vi "Facade.vi"(0 "Data In":T38, 2 "Display State In":T11, 3 "Container State":T37) -> (6 "Data Out":T38, 7 "Display State Out":T11, 8 "Action":T10)   [LabVIEW 2020, in "3DPC_SurfacePlot.xctl"]
uses:
  <vilib>/Native 3D Graph/xcontrol/3DPC_SurfacePlot.xctl
  <vilib>/Native 3D Graph/xcontrol/Data.ctl
  <vilib>/Native 3D Graph/classes/Base Datatype.lvclass
  <vilib>/_xctls/Container State.ctl
  <vilib>/Native 3D Graph/xcontrol/State.ctl
  <vilib>/Native 3D Graph/typedefs/prop_graph.ctl
  <vilib>/Native 3D Graph/typedefs/all_non_graph_prop.ctl
  <vilib>/Native 3D Graph/typedefs/prop_plot_all_array.ctl
  <vilib>/Native 3D Graph/typedefs/prop_plot_all.ctl
  <vilib>/Native 3D Graph/typedefs/prop_plot_projection.ctl
  <vilib>/Native 3D Graph/typedefs/prop_plot_surface.ctl
  <vilib>/Native 3D Graph/typedefs/prop_plot_contour.ctl
  <vilib>/Native 3D Graph/typedefs/prop_plot_normal.ctl
  <vilib>/Native 3D Graph/typedefs/prop_plot_point_line.ctl
  <vilib>/Native 3D Graph/typedefs/prop_value_pair_all.ctl
  <vilib>/Native 3D Graph/typedefs/prop_value_pair_1d.ctl
  <vilib>/Native 3D Graph/typedefs/prop_axes_all.ctl
  <vilib>/Native 3D Graph/typedefs/prop_axes_grid.ctl
  <vilib>/Native 3D Graph/typedefs/prop_axes_ticks.ctl
  <vilib>/Native 3D Graph/typedefs/range_cluster.ctl
  <vilib>/Native 3D Graph/typedefs/min_max.ctl
  <vilib>/Native 3D Graph/typedefs/prop_axes_captions.ctl
  <vilib>/Native 3D Graph/typedefs/prop_axes_labels.ctl
  <vilib>/Native 3D Graph/typedefs/prop_axes_autorange.ctl
  <vilib>/Native 3D Graph/typedefs/prop_cursor_all_array.ctl
  <vilib>/Native 3D Graph/typedefs/prop_cursor_point.ctl
  <vilib>/Native 3D Graph/typedefs/prop_cursor_position.ctl
  <vilib>/Native 3D Graph/typedefs/prop_cursor_line.ctl
  <vilib>/Native 3D Graph/typedefs/prop_cursor_plane.ctl
  <vilib>/Native 3D Graph/typedefs/prop_cursor_text.ctl
  <vilib>/Native 3D Graph/typedefs/prop_format.ctl
  <vilib>/Native 3D Graph/typedefs/prop_lighting.ctl
  <vilib>/_xctls/Action.ctl
  <vilib>/Native 3D Graph/xcontrol/Processed Data.ctl
  <vilib>/Native 3D Graph/typedefs/plot_rep_array.ctl
  <vilib>/Native 3D Graph/typedefs/plot_rep.ctl
  <vilib>/Native 3D Graph/typedefs/plot_rep_mesh_data.ctl
  <vilib>/Native 3D Graph/typedefs/prop_axes_merged_array_etc.ctl
  <vilib>/Native 3D Graph/typedefs/prop_axes_merged_array.ctl
  <vilib>/Utility/miscctls.llb/LVRectTypeDef.ctl
  <vilib>/Native 3D Graph/typedefs/track_eye.ctl
  <vilib>/Native 3D Graph/typedefs/vector.ctl
  <vilib>/Native 3D Graph/typedefs/update_scene_all.ctl
  <vilib>/Native 3D Graph/typedefs/update_scene_component.ctl
  <vilib>/Utility/miscctls.llb/LVPoint32TypeDef.ctl
  <vilib>/picture/3D Picture Control/Object/Create Object (name).vi
  <vilib>/_xctls/XControlSupport.lvlib
  <vilib>/picture/3D Picture Control/NI_3D Picture Control.lvlib
panel:
  in  "Last Axis output cluster":T1={"X Merged Array"=[], "Y Merged Array"=[], "Z Merged Array"=[], "Range Min/Max"={"X"={"Min"=0.0, "Max"=0.0}, "Y"={"Min"=0.0, "Max"=0.0}, "Z"={"Min"=0.0, "Max"=0.0}, "Amplitude"={"Min"=-123456.0, "Max"=-123456.0}}}
  in  "String 2":string="Render Window"
  in  "String":string="3D Graph Properties"
  in  "Coord Systems":T5(array[ring])=[enum."Spherical"]
  in  "Dummy":bool=TRUE
  out "Plot processed data out":T6={"Plot Rep Arrays"=[], "Graph Range Min/Max"={"X"={"Min"=0.0, "Max"=-inf}, "Y"={"Min"=0.0, "Max"=-inf}, "Z"={"Min"=inf, "Max"=-inf}, "Amplitude"={"Min"=0.0, "Max"=0.0}}}
  in  "Plot processed data In":T6={"Plot Rep Arrays"=[], "Graph Range Min/Max"={"X"={"Min"=0.0, "Max"=-inf}, "Y"={"Min"=0.0, "Max"=-inf}, "Z"={"Min"=inf, "Max"=-inf}, "Amplitude"={"Min"=0.0, "Max"=0.0}}} caption="Data In"
  out "Hardware Window Refnum":refnum<vi>
  out "3D Picture Control":refnum<vi>(3d-picture)
types:
  T1 = typedef "3DPC_SurfacePlot.xctl/prop_axes_merged_array_etc.ctl" = cluster{"X Merged Array":T2, "Y Merged Array":T2, "Z Merged Array":T2, "Range Min/Max":T3}
  T2 = typedef "3DPC_SurfacePlot.xctl/prop_axes_merged_array.ctl" = cluster{"Show Tick":bool, "Show Line":bool, "Interval":sgl, "Name":string}[]
  T3 = typedef "3DPC_SurfacePlot.xctl/range_cluster.ctl" = cluster{"X":T4, "Y":T4, "Z":T4, "Amplitude":T4}
  T4 = typedef "3DPC_SurfacePlot.xctl/min_max.ctl" = cluster{"Min":sgl, "Max":sgl}
  T5 = enum16{"Cartesian", "Cylindrical", "Spherical"}[]
  T6 = typedef "Processed Data.ctl" = cluster{"Plot Rep Arrays":T7, "Graph Range Min/Max":T3}
  T7 = typedef "3DPC_SurfacePlot.xctl/plot_rep_array.ctl" = T8[]
  T8 = typedef "3DPC_SurfacePlot.xctl/plot_rep.ctl" = cluster{"Plot ID":i32, "Plot Range Min/Max Out":T3, "Mesh Data":T9}
  T9 = typedef "3DPC_SurfacePlot.xctl/plot_rep_mesh_data.ctl" = cluster{"Index Array":u32[], "Normal Array":cluster{"X":sgl, "Y":sgl, "Z":sgl}[], "Vertex Array":cluster{"X":sgl, "Y":sgl, "Z":sgl}[], "Draw Mode":enum16{"Points", "Lines", "Line Strip", "Line Loop", "Triangles", "Triangle Strip", "Triangle Fan", "Quads", "Quad Strip", "Polygon"}, "Coordinate System":enum16{"Cartesian", "Cylindrical", "Spherical"}, "Color Index Array":i32[]}
  T10 = typedef "XControlSupport.lvlib/Action.ctl" = cluster{"Data Changed?":bool, "State Changed?":bool, "Action Name":string}
  T11 = typedef "3DPC_SurfacePlot.xctl/State.ctl" = cluster{"Graph Properties":T12, "Plot/Axes/Cursor Properties":T13, "Active Plot":i32, "Active Axis":i32, "Active Cursor":i32, "Disable Updates":bool}
  T12 = typedef "3DPC_SurfacePlot.xctl/prop_graph.ctl" = cluster{"Projection Mode":enum16{"Orthographic", "Perspective"}, "View Direction":enum32{"Towards X-Y Plane", "Towards Y-Z Plane", "Towards X-Z Plane", "User Define"}, "Plot Area Color":u32, "Fast Draw":bool, "X-Y":bool, "Y-Z":bool, "X-Z":bool, "Lighting":bool, "Refnum Queue":refnum<queue>}
  T13 = typedef "3DPC_SurfacePlot.xctl/all_non_graph_prop.ctl" = cluster{"Plot Properties Array":T14, "Value Pair Properties":T21, "Axes Properties":T23, "Cursor Properties Array":T29, "Format strings":T35, "Lighting Properties":T36, "Lights":cluster{"Position":cluster{"X":sgl, "Y":sgl, "Z":sgl}, "Direction":cluster{"X":sgl, "Y":sgl, "Z":sgl}}[]}
  T14 = typedef "3DPC_SurfacePlot.xctl/prop_plot_all_array.ctl" = T15[]
  T15 = typedef "3DPC_SurfacePlot.xctl/prop_plot_all.ctl" = cluster{"Projection Properties":T16, "Surface Properties":T17, "Contour Properties":T18, "Normal Properties":T19, "Points/Lines Properties":T20, "Plot ID":i32, "Coordinate System":enum16{"Cartesian", "Cylindrical", "Spherical"}}
  T16 = typedef "3DPC_SurfacePlot.xctl/prop_plot_projection.ctl" = cluster{"Draw XY":bool, "Draw YZ":bool, "Draw XZ":bool}
  T17 = typedef "3DPC_SurfacePlot.xctl/prop_plot_surface.ctl" = cluster{"Draw surface":bool, "Opacity":dbl, "Shading":bool, "Specular":i32, "Color Map":cluster{dbl, u32}[], "Interpolate Color":bool, "Absolute Colormap":bool}
  T18 = typedef "3DPC_SurfacePlot.xctl/prop_plot_contour.ctl" = cluster{"Contour color":u32, "Axis":enum16{"X", "Y", "Z"}, "Draw contour":bool, "Antialias":bool, "Line Width":sgl, "Contour Line Style":enum16{"Solid", "Dash", "Dot", "Dash Dot"}, "Mode":enum16{"Levels", "Intervals", "Level List"}, "Levels":sgl, "Intervals":sgl, "Anchored At":sgl, "Anchored":bool, "Level List":dbl[]}
  T19 = typedef "3DPC_SurfacePlot.xctl/prop_plot_normal.ctl" = cluster{"Normal color":u32, "Normal Length":sgl, "Normal Width":sgl, "Draw Normal":bool, "Antialiasing":bool}
  T20 = typedef "3DPC_SurfacePlot.xctl/prop_plot_point_line.ctl" = cluster{"Color":u32, "Antialiasing":bool, "Point Size":sgl, "Points / Lines":enum16{"None", "Points", "Lines", "Both"}, "Point Style":enum16{"Point", "EmptySquare", "Asterisk", "Diamond", "EmptyCircle", "Circle", "X"}, "Line Style":enum16{"Solid", "Dash", "Dot", "Dash Dot"}, "Line Width":sgl}
  T21 = typedef "3DPC_SurfacePlot.xctl/prop_value_pair_all.ctl" = cluster{"X Value Pairs":cluster{"Data Array":cluster{"Value":sgl, "Index":i32, "Name":string}[], "Show ticks":bool, "Show grid lines":bool, "Labels":enum16{"Value", "None", "Name"}}, "Y Value Pairs":T22, "Z Value Pairs":T22}
  T22 = typedef "3DPC_SurfacePlot.xctl/prop_value_pair_1d.ctl" = cluster{"Data Array":cluster{"Value":sgl, "Index":i32, "Name":string}[], "Show ticks":bool, "Show grid lines":bool, "Labels":enum16{"Value", "None", "Name"}}
  T23 = typedef "3DPC_SurfacePlot.xctl/prop_axes_all.ctl" = cluster{"Grid  Properties":T24, "Ticks Properties":T25, "from/to cluster":T3, "Caption Properties":T26, "Labels Properties":T27, "Auto Range On":T28}
  T24 = typedef "3DPC_SurfacePlot.xctl/prop_axes_grid.ctl" = cluster{"Grid Visible":cluster{"Draw X-grid":bool, "Draw Y-grid":bool, "Draw Z-grid":bool}, "Grid Color":cluster{"Color X":u32, "Color Y":u32, "Color Z":u32}}
  T25 = typedef "3DPC_SurfacePlot.xctl/prop_axes_ticks.ctl" = cluster{"Minor Count":cluster{"X":i32, "Y":i32, "Z":i32}, "Major Count":cluster{"X":i32, "Y":i32, "Z":i32}, "Major Ticks Visible":cluster{"X":bool, "Y":bool, "Z":bool}, "Minor Ticks Visible":cluster{"X":bool, "Y":bool, "Z":bool}, "Tick Color":cluster{"Color X":u32, "Color Y":u32, "Color Z":u32}}
  T26 = typedef "3DPC_SurfacePlot.xctl/prop_axes_captions.ctl" = cluster{"Show Captions":cluster{"Show X Caption":bool, "Show Z Caption":bool, "Show Y Caption":bool, "Show Opposite X Caption":bool, "Show Opposite Y Caption":bool, "Show Opposite Z Caption":bool}, "Captions":cluster{"Caption X":string, "Caption Y":string, "Caption Z":string}, "Caption Color":cluster{"Color X":u32, "Color Y":u32, "Color Z":u32}, "Caption Font Size":cluster{"Font Size X":i16, "Font Size Y":i16, "Font Size Z":i16}}
  T27 = typedef "3DPC_SurfacePlot.xctl/prop_axes_labels.ctl" = cluster{"Label Visible":cluster{"Show X Labels":bool, "Show Y Labels":bool, "Show Z Labels":bool, "Show Opposite X Labels":bool, "Show Opposite Y Labels":bool, "Show Opposite Z Labels":bool}, "Label Color":cluster{"Color X":u32, "Color Y":u32, "Color Z":u32}, "Label Font Size":cluster{"Font Size X":i16, "Font Size Y":i16, "Font Size Z":i16}}
  T28 = typedef "3DPC_SurfacePlot.xctl/prop_axes_autorange.ctl" = cluster{"X":bool, "Y":bool, "Z":bool}
  T29 = typedef "3DPC_SurfacePlot.xctl/prop_cursor_all_array.ctl" = cluster{"Cursor Visible":bool, "Cursor Enable":bool, "Cursor Point":T30, "Cursor Position":T31, "Cursor Line":T32, "Cursor Plane":T33, "Cursor Name":string, "Cursor Text":T34}[]
  T30 = typedef "3DPC_SurfacePlot.xctl/prop_cursor_point.ctl" = cluster{"Point Color":u32, "Point Size":dbl, "Point Visible":bool}
  T31 = typedef "3DPC_SurfacePlot.xctl/prop_cursor_position.ctl" = cluster{"Position X":dbl, "Position Y":dbl, "Position Z":dbl, "Position Snap To":enum16{"Fixed", "Nearest Plot", "Snap to Plot"}, "Polsition Pick Plot":u16, "Position Column":i32, "Position Row":i32}
  T32 = typedef "3DPC_SurfacePlot.xctl/prop_cursor_line.ctl" = cluster{"Line Color":u32, "Line Width":dbl, "Line Visible":bool}
  T33 = typedef "3DPC_SurfacePlot.xctl/prop_cursor_plane.ctl" = cluster{"Plane Opacity":dbl, "Plane Color":u32, "Plane YZ":bool, "Plane XZ":bool, "Plane XY":bool}
  T34 = typedef "3DPC_SurfacePlot.xctl/prop_cursor_text.ctl" = cluster{"Cursor Name":string, "Font Size":i32, "Show Position":bool, "Show Name":bool, "Text Color":u32, "Back Color":u32, "Opacity":dbl}
  T35 = typedef "3DPC_SurfacePlot.xctl/prop_format.ctl" = cluster{"XAxis":string, "YAxis":string, "ZAxis":string}
  T36 = typedef "3DPC_SurfacePlot.xctl/prop_lighting.ctl" = cluster{"Brightness":i32, "Focus":dbl, "Linear Attenuation":dbl, "Quadratic Attenuation":dbl}
  T37 = typedef "XControlSupport.lvlib/Container State.ctl" = cluster{"Indicator?":bool, "Run Mode?":bool, " Refnum":refnum<vi>}
  T38 = typedef "3DPC_SurfacePlot.xctl/Data.ctl" = refnum<class "Base Datatype.lvclass">[]
  T39 = typedef "3DPC_SurfacePlot.xctl/track_eye.ctl" = cluster{"Forward Vect":T40, "Up Vect":T40}
  T40 = typedef "3DPC_SurfacePlot.xctl/vector.ctl" = cluster{"X":sgl, "Y":sgl, "Z":sgl}
  T41 = typedef "LVRectTypeDef.ctl" = cluster{"Left":i16, "Top":i16, "Right":i16, "Bottom":i16}
  T42 = enum16{"Open", "Minimized", "Maximized", "Hidden"}
  T43 = typedef "3DPC_SurfacePlot.xctl/update_scene_all.ctl" = cluster{"Update Plot":T44, "Update Grid":T44, "Update Cursor":T44, "Update Fast Draw":T44}
  T44 = typedef "3DPC_SurfacePlot.xctl/update_scene_component.ctl" = enum16{"Update & Add", "Update & Not Add", "Remove ", "Nothing", "Add"}
  T45 = enum32{"Towards X-Y Plane", "Towards Y-Z Plane", "Towards X-Z Plane", "User Define"}
  T46 = typedef "LVPoint32TypeDef.ctl" = cluster{"Horizontal":i32, "Vertical":i32}
  T47 = cluster{"Real Matrix Element":dbl, "Real Matrix Element":dbl, "Real Matrix Element":dbl}[]
  T48 = cluster{"Left":sgl, "Left":sgl, "Left":sgl, "Left":sgl, "Left":sgl, "Left":sgl}
  T49 = enum16{"None", "Spherical", "Flying", "Oriented"}
  T50 = cluster{"Position":cluster{"X":sgl, "Y":sgl, "Z":sgl}, "Direction":cluster{"X":sgl, "Y":sgl, "Z":sgl}}[]
  T51 = typedef "LVBoundsTypeDef.ctl" = cluster{"Width":u32, "Height":u32}
  T52 = typedef "3DPC_SurfacePlot.xctl/state_scene_objects.ctl" = cluster{"Root":refnum<vi>, "Fast Draw Scene Object":refnum<vi>, "Plot Scene Object":refnum<vi>, "Axes Scene Object":refnum<vi>, "Cursor Scene Object":refnum<vi>, "PL Scene Object":refnum<vi>}
  T53 = cluster{"Cursor Visible":bool, "Cursor Enable":bool, "Cursor Point":T30, "Cursor Position":T31, "Cursor Line":T32, "Cursor Plane":T33, "Cursor Name":string, "Cursor Text":T34}
  T54 = typedef "LV3DPointTypeDef.ctl" = cluster{"X":sgl, "Y":sgl, "Z":sgl}
  T55 = cluster{"X":cluster{"Min":bool, "Max":bool}, "Y":cluster{"Min":bool, "Max":bool}, "Z":cluster{"Min":bool, "Max":bool}, "Amplitude":cluster{"Min":bool, "Max":bool}}
  T56 = cluster{"Shift":bool, "Ctrl":bool, "Alt":bool, "Cmd":bool, "Opt":bool}
  T57 = cluster{"Position X":dbl, "Position Y":dbl, "Position Z":dbl}
  T58 = cluster{"Position X":dbl, "Position Y":dbl, "Position Z":dbl}[]
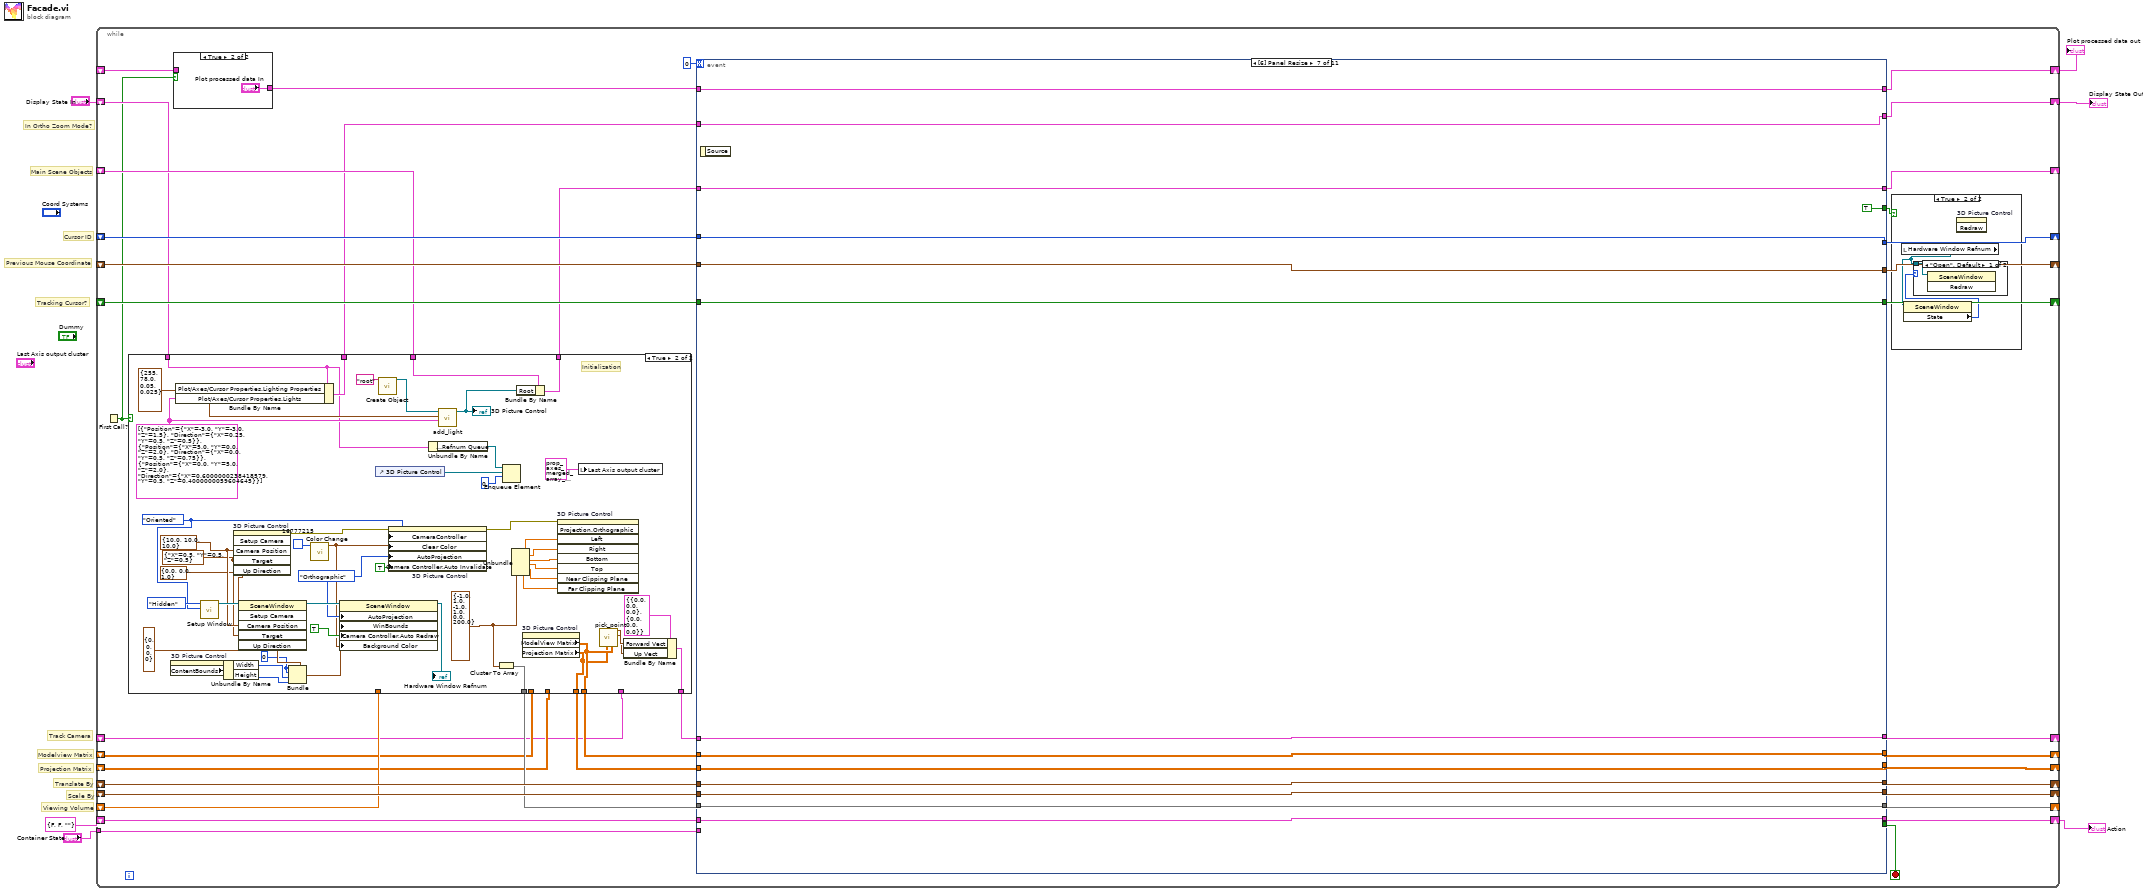
[diagram p0: block diagram]
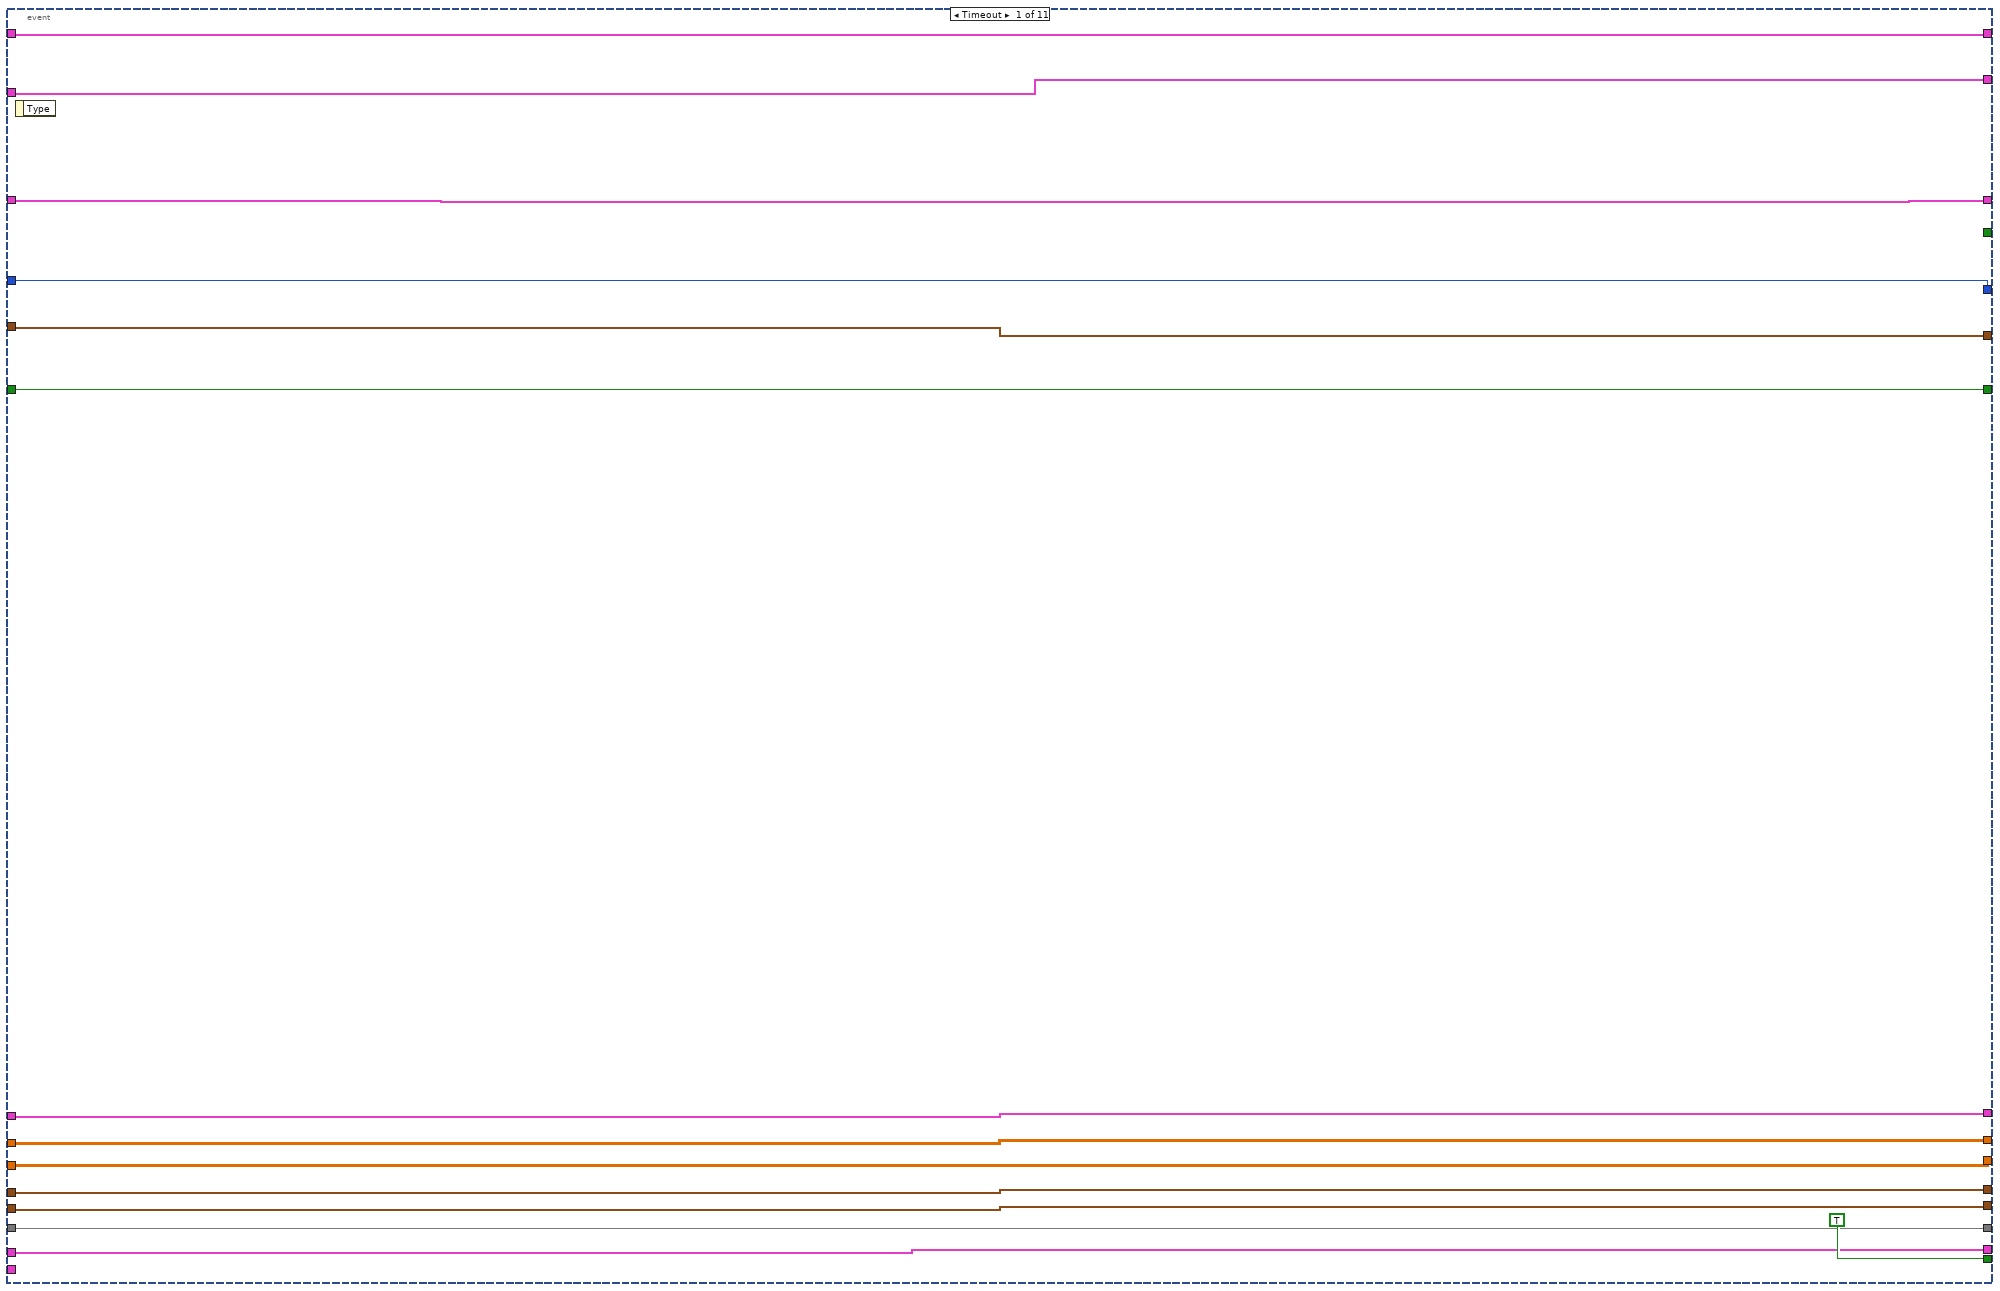
[diagram p6: hidden frame]
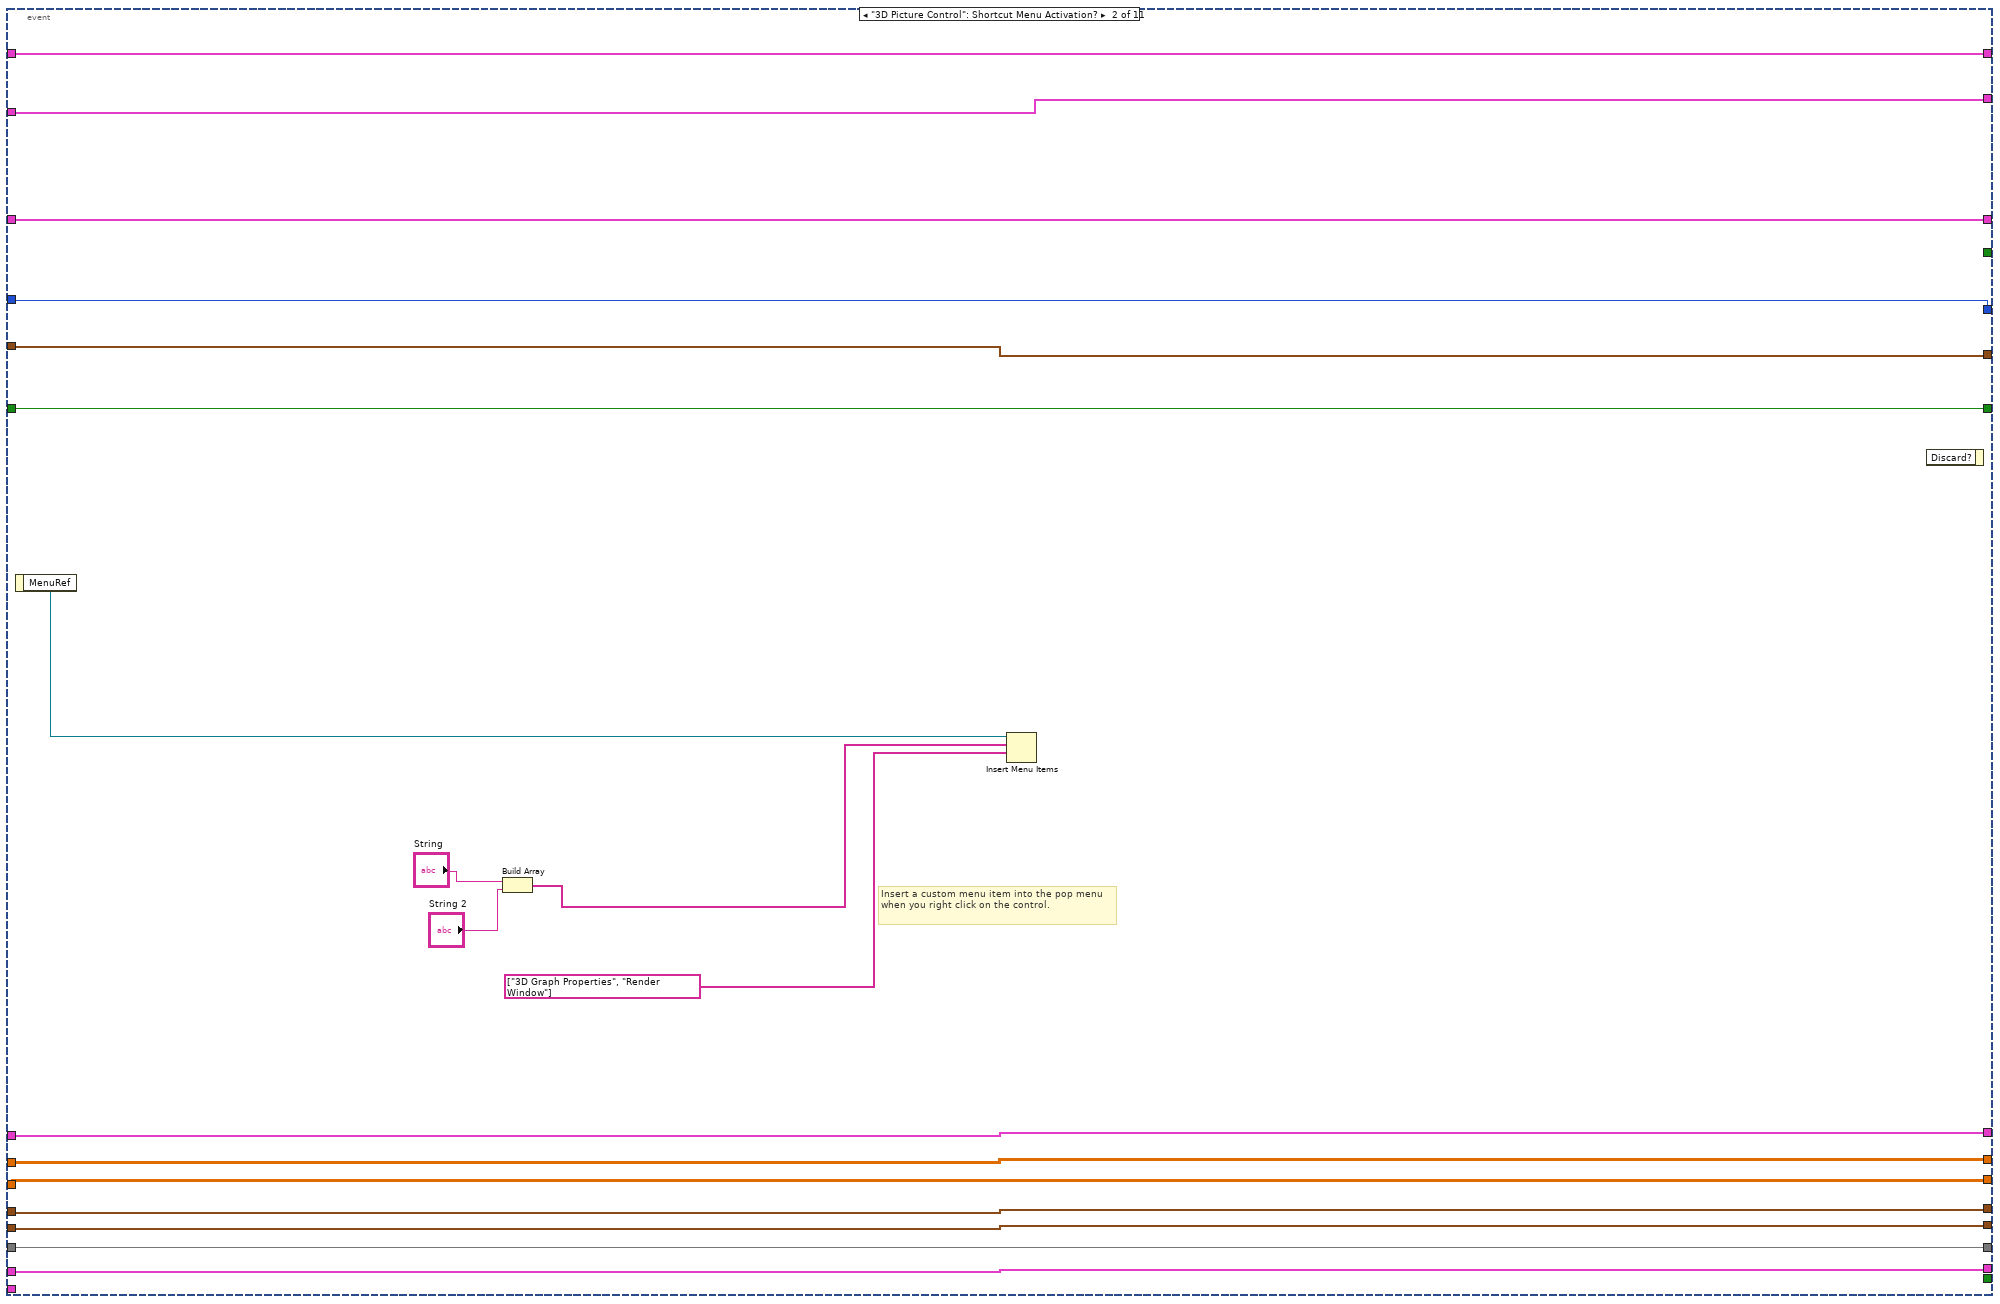
[diagram p7: hidden frame]
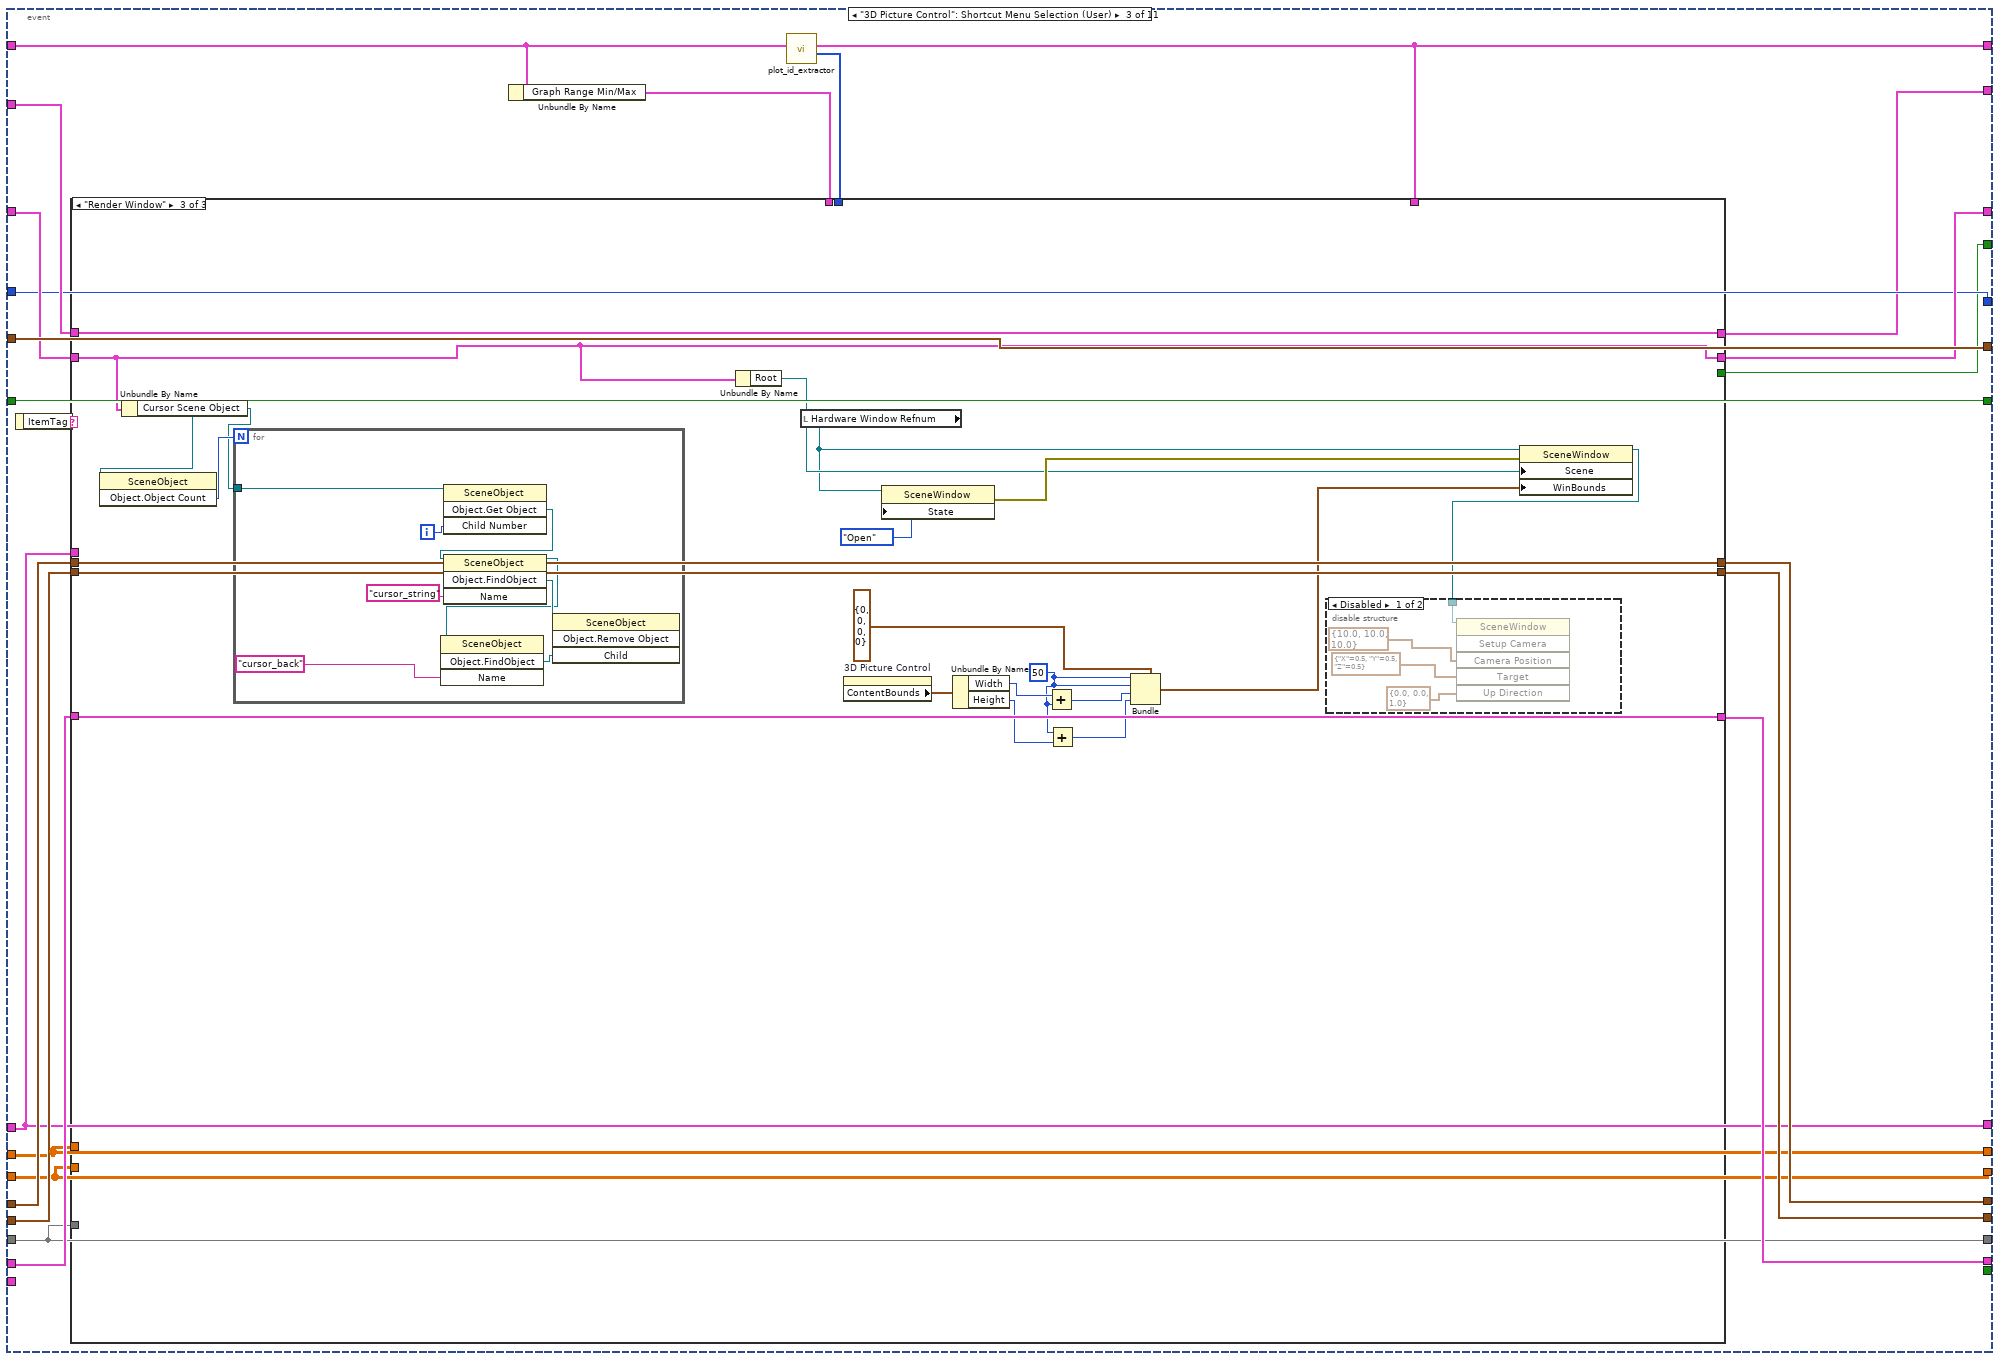
[diagram p8: hidden frame]
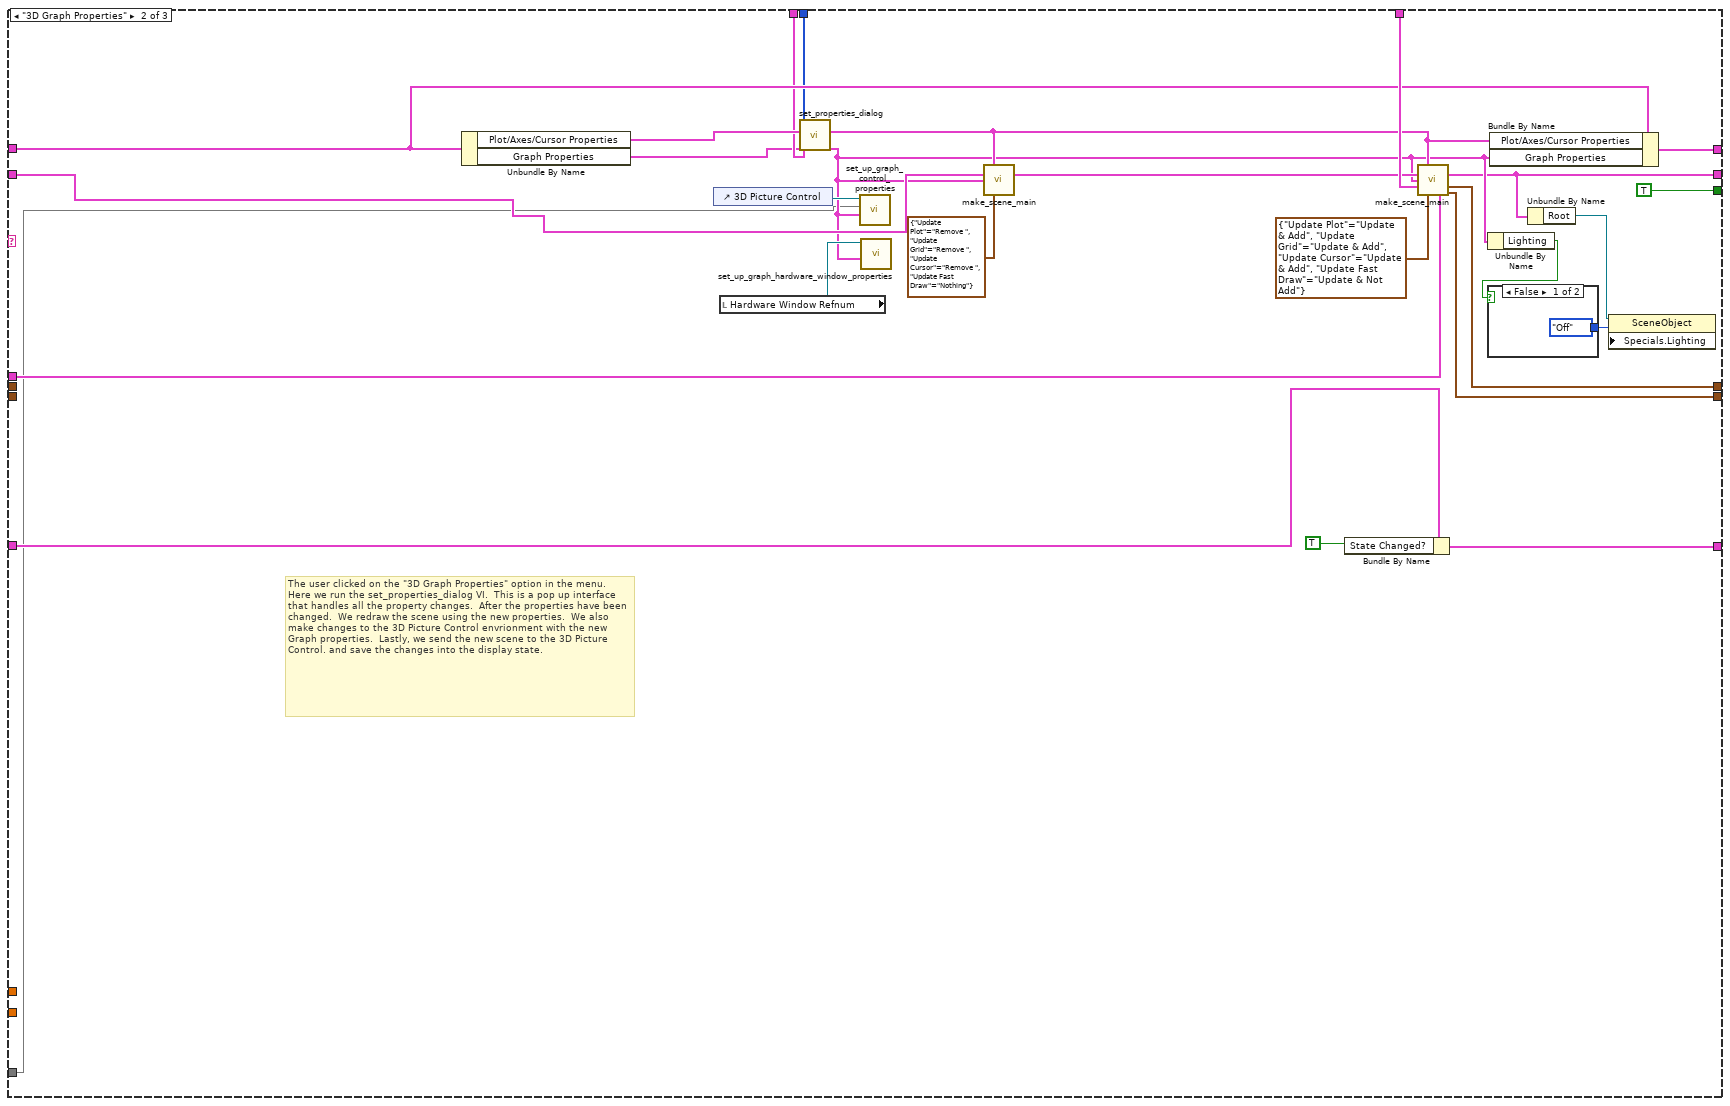
[diagram p10: hidden frame]
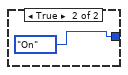
[diagram p11: hidden frame]
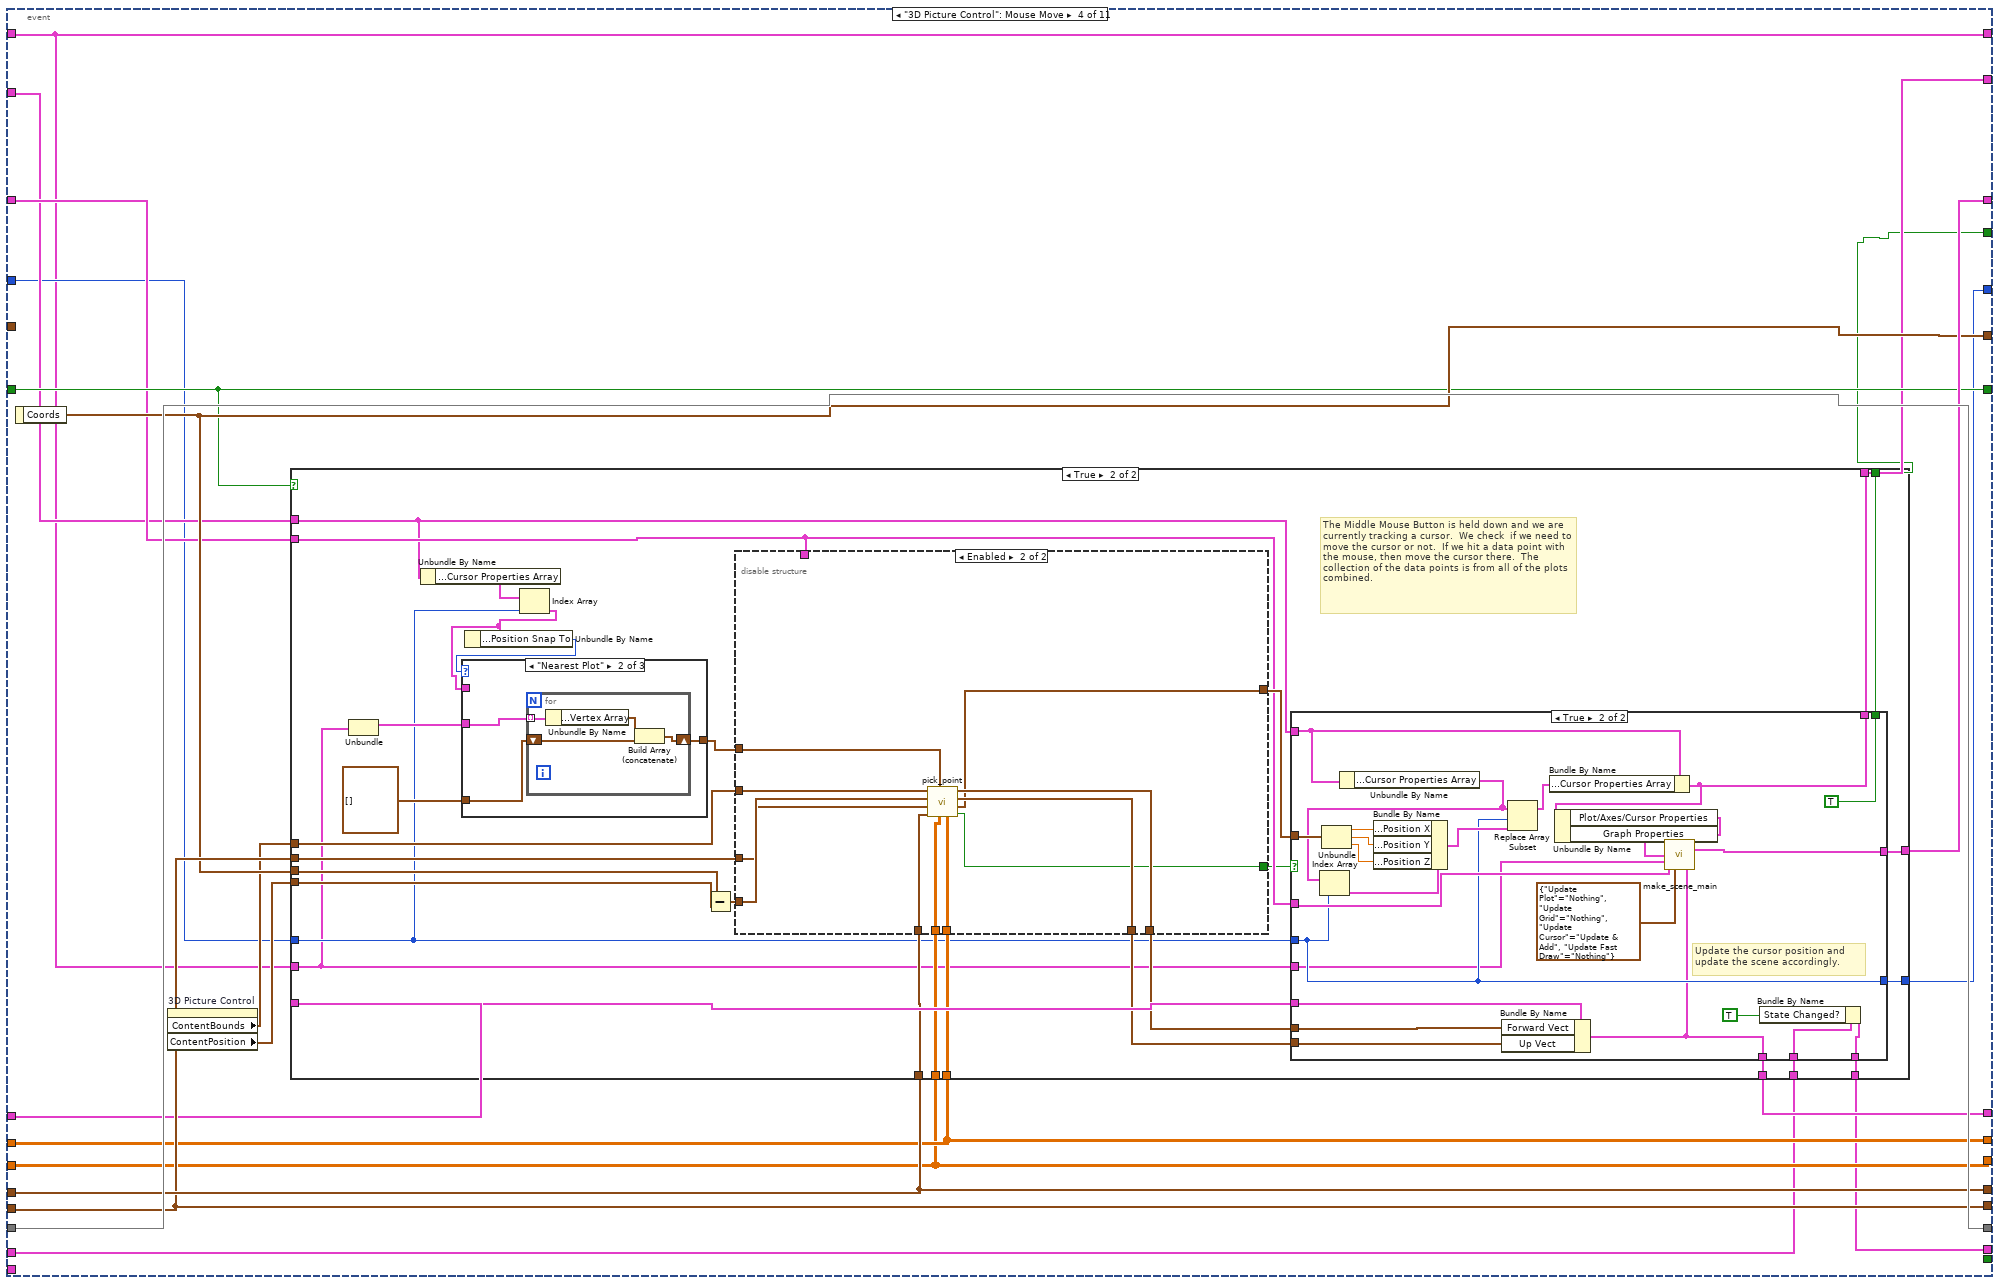
[diagram p13: hidden frame]
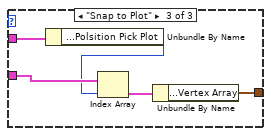
[diagram p16: hidden frame]
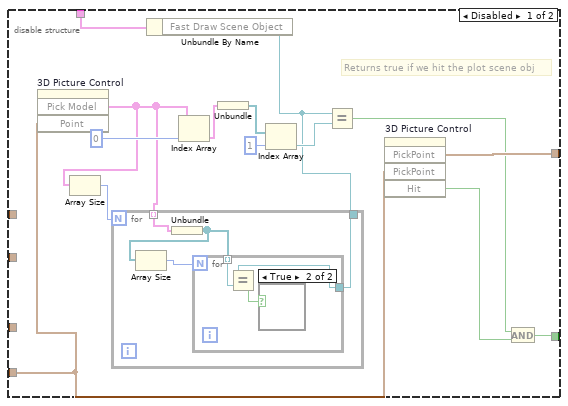
[diagram p17: hidden frame]
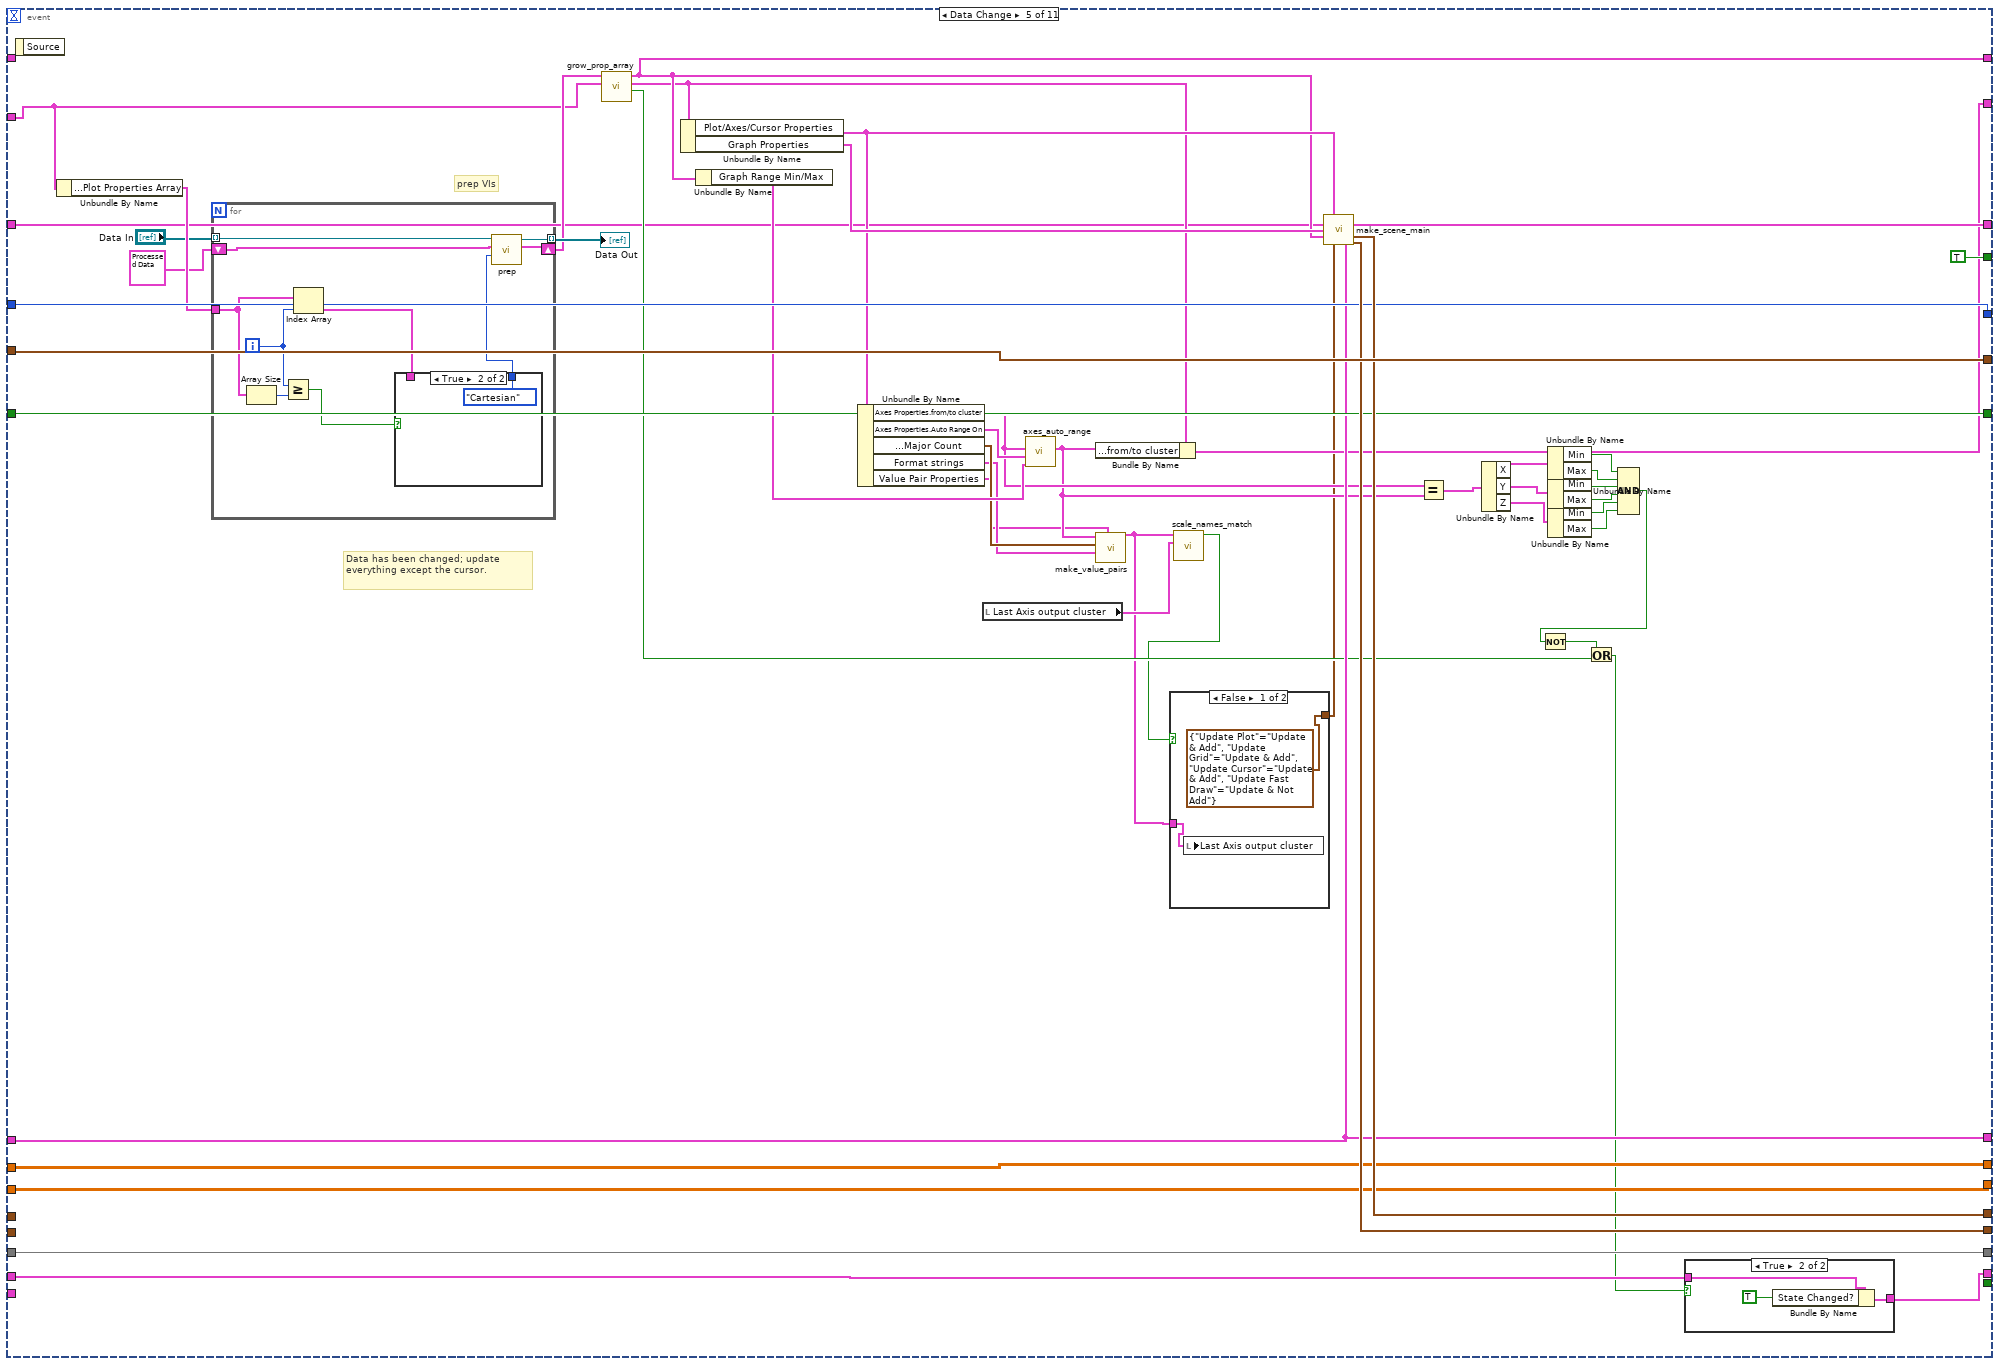
[diagram p20: hidden frame]
diagram:
  # "Viewing Volume"
  # "Main Scene Objects"
  # "Cursor ID"
  # "Scale By"
  # "Translate By"
  # "Projection Matrix"
  # "Modelview Matrix"
  # "Track Camera"
  # "Tracking Cursor?"
  # "In Ortho Zoom Mode?"
  # "Previous Mouse Coordinate"
  n1 = while {
    shift-right: [w25] -> w3
    shift-left: "Display State In" -> [w18]
    tunnel: "Container State" -> [w42]
    shift-right: [w16] -> w6
    shift-left: _ -> [w14]
    shift-right: [w40] -> w4
    shift-left: T10 {"Data Changed?"=FALSE, "State Changed?"=FALSE, "Action Name"=""} ("Action") -> [w41]
    shift-right: [w38] -> _
    shift-left: _ -> [w39]
    shift-right: [w37] -> _
    shift-left: _ -> [w21]
    shift-right: [w36] -> _
    shift-left: _ -> [w24]
    shift-right: [w26] -> _
    shift-left: _ -> [w28]
    shift-right: [w31] -> _
    shift-left: _ -> [w8]
    shift-right: [w30] -> _
    shift-left: _ -> [w12]
    shift-right: [w35] -> _
    shift-left: _ -> [w33]
    shift-right: [w34] -> _
    shift-left: _ -> [w32]
    shift-right: [w27] -> _
    shift-left: _ -> [w29]
    shift-right: [w19] -> _
    shift-left: _ -> [w10]
    stop <- w44 stop-if-true
    n2 = First Call?() -> (First Call?: T/F=w15:bool)
    n3 = case shown="True" w15 {
      tunnel: w24 -> [w54 w101]
      tunnel: [w54 w102] -> w23
      tunnel: w21 -> [w55 _]
      tunnel: [w55 w97] -> w20
      tunnel: w18 -> [w53 w70]
      tunnel: [w53 w96] -> w17
      tunnel: w12 -> [w52 _]
      tunnel: w10 -> [w51 _]
      tunnel: w8 -> [w50 _]
      tunnel: [w52 w62] -> w11
      tunnel: [w51 w61] -> w9
      tunnel: [w50 w57] -> w7
      frame False {
      }
      frame True {
        w76 = T48 {"Left"=-1.0, "Left"=1.0, "Left"=-1.0, "Left"=1.0, "Left"=0.0, "Left"=200.0} ("output cluster")
        w75 = T49."Oriented" ("Camera Controller:Type")
        w80 = i16 0 ("Left")
        w94 = T50 [{"Position"={"X"=-3.0, "Y"=-3.0, "Z"=1.5}, "Direction"={"X"=0.25, "Y"=0.5, "Z"=0.5}}, {"Position"={"X"=5.0, "Y"=0.0, "Z"=2.0}, "Direction"={"X"=0.0, "Y"=0.5, "Z"=0.75}}, {"Position"={"X"=0.0, "Y"=5.0, "Z"=2.0}, "Direction"={"X"=0.6, "Y"=0.5, "Z"=0.4}}] ("Plot/Axes/Cursor Properties.Lights")
        w95 = T36 {"Brightness"=255, "Focus"=78.0, "Linear Attenuation"=0.05, "Quadratic Attenuation"=0.025} ("Plot/Axes/Cursor Properties.Lighting Properties")
        w89 = cluster{"Z":sgl, "Y":sgl, "X":sgl} {"Z"=0.0, "Y"=0.0, "X"=1.0}
        w90 = cluster{"X":sgl, "Y":sgl, "Z":sgl} {"X"=0.5, "Y"=0.5, "Z"=0.5} ("Target")
        w91 = cluster{"X":sgl, "Y":sgl, "Z":sgl} {"X"=10.0, "Y"=10.0, "Z"=10.0} ("Up Direction")
        w87 = enum16{"None", "Perspective", "Orthographic"}."Orthographic" ("Automatic Projection Mode")
        # "Initialization"
        n4 = property on="3D Picture Control" class="SceneGraphDisp (strict)"() -> ("ContentBounds"=w84:T51)  [unwired: 2 in, 2 out]
        n5 = Bundle By Name(cluster=w70, "Plot/Axes/Cursor Properties.Lighting Properties"=w95, "Plot/Axes/Cursor Properties.Lights"=w94) -> (w96:T11)
        n6 = call <vilib>:"Setup Window.vi"("Camera Controller"=w75, "Window State"=T42."Hidden") -> ("New Window Refnum"=w93:refnum<vi>)  [unwired: 1 in, 8 out]
        n7 = Unbundle By Name(w84) -> ("Width"=w82:u32, "Height"=w81:u32)
        n8 = invoke on="3D Picture Control" class="SceneGraphDisp (strict)" method="Setup Camera"("Camera Position"=w91, "Target"=w90, "Up Direction"=w89) -> (error out=w74:errorcluster)  [unwired: 3 in, 5 out]
        n9 = invoke class="SceneWindow" method="Setup Camera"(reference=w93, "Camera Position"=w91, "Target"=w90, "Up Direction"=w89) -> (reference out=w88:refnum<vi>)  [unwired: 2 in, 5 out]
        n10 = Bundle(cluster=T41 {"Left"=0, "Top"=0, "Right"=0, "Bottom"=0} ("Window Bounds"), "Left"=w80, "Top"=w80, "Right"=w82, "Bottom"=w81) -> (w79:T41)
        n11 = call <vilib>:"Color Change.vi"("Color"=u32 16777215) -> ("RGBA"=w85:cluster{"R":sgl, "G":sgl, "B":sgl, "A":sgl})  [unwired: 1 in, 9 out]
        n12 = property class="SceneWindow"(reference=w88, "AutoProjection"=w87, "WinBounds"=w79, "Camera Controller.Auto Redraw"=TRUE ("Camera Controller:Auto Redraw"), "Background Color"=w85) -> (reference out=→"Hardware Window Refnum":refnum<vi>)  [unwired: 1 in, 1 out]
        n13 = control-ref of="3D Picture Control"() -> (w73:refnum<vi>)
        n14 = call-poly <vilib>:"Create Object.vi"("Name"="root") -> ("Scene:New Object"=w103:refnum<vi>)  [unwired: 9 in, 1 out]
        n15 = property on="3D Picture Control" class="SceneGraphDisp (strict)"(error in=w74, "CameraController"=w75, "Clear Color"=w85, "AutoProjection"=w87, "Camera Controller.Auto Invalidate"=TRUE ("Camera Controller:Auto Invalidate")) -> (error out=w77:errorcluster)  [unwired: 1 in, 1 out]
        n16 = Unbundle By Name(w70) -> ("Graph Properties.Refnum Queue"=w72:refnum<queue>)
        n17 = call <vilib>:"add_light.vi"("Lights"=w94, "Lighting Properties"=w95, "Scene:New Object"=w103) -> ("Scene:New Object 2"=w100:refnum<vi>)  [unwired: 8 out]
        "3D Picture Control" <- w100
        n18 = Cluster To Array(cluster=w76) -> (array=w97:sgl[])
        n19 = Enqueue Element(queue=w72, element=w73, timeout in ms (-1)=0) -> ()  [unwired: 1 in, 3 out]
        n20 = Unbundle(w76) -> ("Left"=w69:sgl, "Left"=w68:sgl, "Left"=w67:sgl, "Left"=w66:sgl, "Left"=w65:sgl, "Left"=w64:sgl)
        n21 = Bundle By Name(cluster=w101, "Root"=w100) -> (w102:T52)
        n22 = property on="3D Picture Control" class="SceneGraphDisp (strict)"() -> ("ModelView Matrix"=w62:sgl[][], "Projection Matrix"=w61:sgl[][])  [unwired: 2 in, 2 out]
        n23 = invoke on="3D Picture Control" class="SceneGraphDisp (strict)" method="Projection.Orthographic"(error in=w77, "Left"=w69, "Right"=w68, "Bottom"=w67, "Top"=w66, "Near Clipping Plane"=w65, "Far Clipping Plane"=w64) -> ()  [unwired: 2 in, 9 out]
        n24 = local write "Last Axis output cluster"(T1 {"X Merged Array"=[], "Y Merged Array"=[], "Z Merged Array"=[], "Range Min/Max"={"X"={"Min"=0.0, "Max"=0.0}, "Y"={"Min"=0.0, "Max"=0.0}, "Z"={"Min"=0.0, "Max"=0.0}, "Amplitude"={"Min"=0.0, "Max"=0.0}}} ("Last Axis output cluster")) -> ()
        n25 = call <vilib>:"pick_point.vi"("Modelview Matrix"=w62, "Projection Matrix"=w61) -> ("Up Vect"=w58:T40, "Forward Vect"=w59:T40)  [unwired: 5 in, 3 out]
        n26 = Bundle By Name(cluster=T39 {"Forward Vect"={"X"=0.0, "Y"=0.0, "Z"=0.0}, "Up Vect"={"X"=0.0, "Y"=0.0, "Z"=0.0}} ("Track Eye"), "Forward Vect"=w59, "Up Vect"=w58) -> (w57:T39)
      }
    }
    n27 = case shown="True" w15 {
      tunnel: w14 -> [w45 _]
      tunnel: [w45 "Plot processed data In"] -> w13
      frame False {
      }
      frame True {
      }
    }
    n28 = event shown="[6] Panel Resize" {
      selector: _ -> [_ _ _ _ _ _ _ _ _ _ _]
      dyn-events: _ -> [_ _ _ _ _ _ _ _ _ _ _]
      timeout: 0 -> [_ _ _ _ _ _ _ _ _ _ _]
      tunnel: w17 -> [w106 w123 w157 w230 w371 w438 w604 w635 w659 w734 w748]
      tunnel: [TRUE _ _ _ _ _ _ _ _ _ _] -> w44
      tunnel: w42 -> [_ _ _ _ _ _ _ _ _ w746 w760]
      tunnel: w13 -> [w116 w135 w140 w228 _ w435 w610 w639 w649 w745 w759]
      tunnel: [w116 w135 w142 w228 w370 w435 w610 w639 w648 w745 w759] -> w16
      tunnel: [w104 w134 w156 w226 w386 w426 w616 w644 w662 w744 w758] -> w40
      tunnel: w41 -> [w104 w134 w155 w227 w387 w427 w616 w644 w662 w744 w758]
      tunnel: w39 -> [w115 w133 w154 _ w404 _ w606 _ w666 w743 w757]
      tunnel: [w115 w133 w154 w240 w404 w441 w606 T46 {"Horizontal"=0, "Vertical"=0} ("Coords") w666 w743 w757] -> w38
      tunnel: w20 -> [w108 w132 w136 w245 w403 w450 w603 w643 w650 w742 w756]
      tunnel: [w108 w132 w136 w245 w403 w450 w603 w643 w650 w742 w756] -> w37
      tunnel: w23 -> [w107 w131 w153 w232 w355 w436 w609 w640 w657 w741 w755]
      tunnel: [w107 w131 w152 w242 w393 w434 w609 w630 w656 w741 w755] -> w36
      tunnel: w7 -> [w114 w130 w147 w233 w397 w449 w611 _ w655 w738 w754]
      tunnel: [w112 w128 w151 w244 w402 w443 w614 w642 w651 w740 w752] -> w35
      tunnel: [w111 w127 w150 w243 w401 w442 w615 w641 w653 w739 w751] -> w34
      tunnel: w33 -> [w112 w128 w149 w244 _ w443 w614 w642 w652 w740 w752]
      tunnel: w32 -> [w111 w127 w148 w243 _ w442 w615 w641 w654 w739 w751]
      tunnel: w11 -> [w113 w129 w138 w235 w400 w444 w612 _ w665 w737 w753]
      tunnel: [w114 w130 w147 w236 w397 w449 w611 w631 w655 w738 w754] -> w31
      tunnel: [w113 w129 w138 w235 w400 w444 w612 w619 w665 w737 w753] -> w30
      tunnel: [w105 w122 w137 w231 w395 w432 w613 w618 w660 w733 w747] -> w19
      tunnel: w29 -> [w110 w126 w146 w229 w399 w448 w607 w638 w664 w736 w750]
      tunnel: w28 -> [w109 w124 w145 w238 w398 w447 w605 _ w663 w735 w749]
      tunnel: [w110 w126 w146 w237 w399 w440 w607 w638 w664 w736 w750] -> w27
      tunnel: [w109 w124 w145 w238 w398 w439 w605 FALSE ("x .and. y?") w663 w735 w749] -> w26
      tunnel: [w106 w123 w144 w234 w389 w428 w604 w635 w659 w734 w748] -> w25
      tunnel: [_ _ w143 w225 TRUE w433 TRUE TRUE TRUE _ _] -> w22
      tunnel: w9 -> [w105 w122 w137 w231 w395 w432 w613 _ w660 w733 w747]
      event Timeout {
        n29 = event-data() -> ()  [unwired: 2 out]
      }
      event "3D Picture Control": Shortcut Menu Activation? {
        # "Insert a custom menu item into the pop menu when you right click on the control."
        n30 = event-data() -> ("MenuRef"=w125:refnum<k9>)  [unwired: 1 out]
        n31 = Build Array("String", "String 2") -> (w118:string[])
        n32 = Insert Menu Items(7:string[] ["3D Graph Properties", "Render Window"] ("item names 2"), 8:w118, 9:w125) -> ()  [unwired: 1 in, 5 out]
        n33 = event-data() -> ()  [unwired: 1 in, 2 out]
      }
      event "3D Picture Control": Shortcut Menu Selection (User) {
        n34 = event-data() -> ("ItemTag"=w158:string)  [unwired: 1 out]
        n35 = Unbundle By Name(w140) -> ("Graph Range Min/Max"=w139:T3)
        n36 = call <vilib>:"plot_id_extractor.vi"("Plot processed data In"=w140) -> ("Plot IDs"=w141:i32[], "Plot processed data Out"=w142:T6)  [unwired: 9 out]
        n37 = case shown="\"Render Window\"" w158 {
          tunnel: w157 -> [w163 w183 w207]
          tunnel: [w163 w182 w207] -> w144
          tunnel: [w162 w190 w210] -> w156
          tunnel: w155 -> [w162 w181 w210]
          tunnel: w142 -> [_ w188 _]
          tunnel: w153 -> [w161 w168 w202]
          tunnel: [w161 w165 w202] -> w152
          tunnel: w147 -> [_ w187 _]
          tunnel: [w160 w186 w208] -> w151
          tunnel: [w159 w185 w209] -> w150
          tunnel: w149 -> [w160 _ w208]
          tunnel: w148 -> [w159 _ w209]
          tunnel: [_ TRUE _] -> w143
          tunnel: w141 -> [_ w174 _]
          tunnel: w139 -> [_ w173 _]
          tunnel: w138 -> [_ _ _]
          tunnel: w137 -> [_ _ _]
          tunnel: w136 -> [_ w164 _]
          frame "False", Default {
          }
          frame "3D Graph Properties" {
            # "The user clicked on the \"3D Graph Properties\" option in the menu.  Here we run the set_properties_dialog VI.  This is a pop up interface that handles all the property changes.  After the properties have been changed.  We redraw the scene using the new properties.  We also make changes to the 3D Picture Control envrionment with the new Graph properties.  Lastly, we send the new scene to the 3D Picture Control. and save the changes into the display state."
            n38 = Unbundle By Name(w183) -> ("Plot/Axes/Cursor Properties"=w184:T13, "Graph Properties"=w167:T12)
            n39 = control-ref of="3D Picture Control"() -> (w180:refnum<vi>)
            n40 = local read "Hardware Window Refnum"() -> (w175:refnum<vi>)
            n41 = call <vilib>:"set_properties_dialog.vi"("Graph Range Min/Max"=w173, "Graph Properties In"=w167, "All Properties"=w184, "Plot IDs"=w174) -> ("Graph Properties Out"=w166:T12, "All Properties Out"=w172:T13)  [unwired: 6 out]
            n42 = call <vilib>:"set_up_graph_control_properties.vi"("Graph Properties"=w166, "viewing volume"=w164, "3D Picture Control Reference"=w180) -> ()  [unwired: 9 out]
            n43 = call <vilib>:"set_up_graph_hardware_window_properties.vi"("Graph Properties"=w166, "Hardware Window Refnum"=w175) -> ()  [unwired: 10 out]
            n44 = call <vilib>:"make_scene_main.vi"("All Properties"=w172, "Scene Objects In"=w168, "Graph Properties"=w166, "Update?"=T43 {"Update Plot"=enum."Remove ", "Update Grid"=enum."Remove ", "Update Cursor"=enum."Remove ", "Update Fast Draw"=enum."Nothing"}) -> ("Scene Objects Out"=w178:T52)  [unwired: 2 in, 9 out]
            n45 = Bundle By Name(cluster=w181, "State Changed?"=TRUE ("Data Changed?")) -> (w190:T10)
            n46 = call <vilib>:"make_scene_main.vi"("All Properties"=w172, "Scene Objects In"=w178, "Graph Properties"=w166, "Plot Processed Data"=w188, "Update?"=T43 {"Update Plot"=enum."Update & Add", "Update Grid"=enum."Update & Add", "Update Cursor"=enum."Update & Add", "Update Fast Draw"=enum."Update & Not Add"}, "Track Eye"=w187) -> ("Scene Objects Out"=w165:T52, "Translate By"=w186:T40, "Scale By"=w185:T40)  [unwired: 7 out]
            n47 = Unbundle By Name(w166) -> ("Lighting"=w171:bool)
            n48 = case shown="False" w171 {
              tunnel: [enum16{"Inherit Value", "Off", "On"}."Off" ("Specials:Lighting") enum16{"Inherit Value", "Off", "On"}."On" ("Specials:Lighting")] -> w170
              frame False {
              }
              frame True {
              }
            }
            n49 = Bundle By Name(cluster=w183, "Plot/Axes/Cursor Properties"=w172, "Graph Properties"=w166) -> (w182:T11)
            n50 = Unbundle By Name(w165) -> ("Root"=w169:refnum<vi>)
            n51 = property class="SceneObject"(reference=w169, "Specials.Lighting"=w170) -> ()  [unwired: 1 in, 2 out]
          }
          frame "Render Window" {
            w196 = i16 50 ("Left")
            n52 = Unbundle By Name(w202) -> ("Cursor Scene Object"=w200:refnum<vi>)
            n53 = invoke class="SceneObject" method="Object.Object Count"(reference=w200) -> ("Child Count"=w201:i32)  [unwired: 2 in, 2 out]
            n54 = for {
              N: w201 -> [_]
              tunnel: w200 -> [w224]
              i -> [w223]
              n55 = invoke class="SceneObject" method="Object.Get Object"(reference=w224, "Child Number"=w223) -> ("Get Child"=w217:refnum<vi>)  [unwired: 2 in, 3 out]
              n56 = invoke class="SceneObject" method="Object.FindObject"(reference=w217, "Name"="cursor_string") -> (reference out=w219:refnum<vi>, "FindObject"=w221:refnum<vi>)  [unwired: 2 in, 2 out]
              n57 = invoke class="SceneObject" method="Object.FindObject"(reference=w219, "Name"="cursor_back") -> ("FindObject"=w222:refnum<vi>)  [unwired: 2 in, 3 out]
              n58 = invoke class="SceneObject" method="Object.Remove Object"(reference=w221, "Child"=w222) -> ()  [unwired: 2 in, 4 out]
            }
            n59 = Unbundle By Name(w202) -> ("Root"=w211:refnum<vi>)
            n60 = local read "Hardware Window Refnum"() -> (w199:refnum<vi>)
            n61 = property on="3D Picture Control" class="SceneGraphDisp (strict)"() -> ("ContentBounds"=w203:T51)  [unwired: 2 in, 2 out]
            n62 = property class="SceneWindow"(reference=w199, "State"=T42."Open" ("Window State")) -> (error out=w212:errorcluster)  [unwired: 1 in, 1 out]
            n63 = Unbundle By Name(w203) -> ("Width"=w198:u32, "Height"=w197:u32)
            n64 = Add(x=w198, y=w196) -> (x+y=w194:u32)
            n65 = Add(x=w196, y=w197) -> (x+y=w195:u32)
            n66 = Bundle(cluster=T41 {"Left"=0, "Top"=0, "Right"=0, "Bottom"=0} ("Window Bounds"), "Left"=w196, "Top"=w196, "Right"=w194, "Bottom"=w195) -> (w204:T41)
            n67 = property class="SceneWindow"(reference=w199, error in=w212, "Scene"=w211, "WinBounds"=w204) -> (reference out=w193:refnum<vi>)  [unwired: 1 out]
            n68 = disable-structure shown="Disabled" {
              disable-tunnel: w193 -> [w216 _]
              frame Disabled {
                n69 = invoke class="SceneWindow" method="Setup Camera"(reference=w216, "Camera Position"=cluster{"X":sgl, "Y":sgl, "Z":sgl} {"X"=10.0, "Y"=10.0, "Z"=10.0} ("Up Direction"), "Target"=cluster{"X":sgl, "Y":sgl, "Z":sgl} {"X"=0.5, "Y"=0.5, "Z"=0.5}, "Up Direction"=cluster{"Z":sgl, "Y":sgl, "X":sgl} {"Z"=0.0, "Y"=0.0, "X"=1.0}) -> ()  [unwired: 2 in, 6 out]
              }
              frame Enabled {
              }
            }
          }
        }
      }
      event "3D Picture Control": Mouse Move {
        n70 = event-data() -> ("Coords"=w240:T46)  [unwired: 1 out]
        n71 = property on="3D Picture Control" class="SceneGraphDisp (strict)"() -> ("ContentBounds"=w239:T51, "ContentPosition"=w241:T46)  [unwired: 2 in, 2 out]
        n72 = case shown="True" w238 {
          tunnel: w239 -> [_ w265]
          tunnel: w241 -> [_ w279]
          tunnel: w240 -> [_ w280]
          tunnel: w243 -> [_ w264]
          tunnel: w244 -> [_ w263]
          tunnel: w232 -> [w250 w270]
          tunnel: [w250 w278] -> w242
          tunnel: w229 -> [w249 w255]
          tunnel: [w249 w277] -> w237
          tunnel: w233 -> [w247 w276]
          tunnel: w228 -> [_ w253]
          tunnel: w230 -> [w248 w256]
          tunnel: [w248 w275] -> w234
          tunnel: [w247 w274] -> w236
          tunnel: w235 -> [_ w266]
          tunnel: [_ w273] -> w225
          tunnel: w231 -> [_ w262]
          tunnel: w227 -> [w246 w252]
          tunnel: [w246 w251] -> w226
          frame False {
          }
          frame True {
            # "The Middle Mouse Button is held down and we are currently tracking a cursor.  We check  if we need to move the cursor or not.  If we hit a data point with the mouse, then move the cursor there.  The collection of the data points is from all of the plots combined."
            n73 = Unbundle(w253) -> ("Plot Rep Arrays"=w257:T7)  [unwired: 1 out]
            n74 = Unbundle By Name(w256) -> ("Plot/Axes/Cursor Properties.Cursor Properties Array"=w259:T29)
            n75 = Index Array(array=w259, index=w255) -> (element=w261:T53)
            n76 = Unbundle By Name(w261) -> ("Cursor Position.Position Snap To"=w260:enum16{"Fixed", "Nearest Plot", "Snap to Plot"})
            n77 = case shown="\"Nearest Plot\"" w260 {
              tunnel: [_ w283 w288] -> w254
              tunnel: w257 -> [_ w282 w291]
              tunnel: cluster{"X":sgl, "Y":sgl, "Z":sgl}[] [] -> [_ w281 _]
              tunnel: w261 -> [_ _ w292]
              frame "Fixed", Default {
              }
              frame "Nearest Plot" {
                n78 = for {
                  tunnel: w282 -> [w287] mode=indexing
                  shift-right: [w284] -> w283
                  shift-left: w281 -> [w285]
                  n79 = Unbundle By Name(w287) -> ("Mesh Data.Vertex Array"=w286:cluster{"X":sgl, "Y":sgl, "Z":sgl}[])
                  n80 = Build Array (concatenate)(w286, w285) -> (w284:cluster{"X":sgl, "Y":sgl, "Z":sgl}[])
                }
              }
              frame "Snap to Plot" {
                n81 = Unbundle By Name(w292) -> ("Cursor Position.Polsition Pick Plot"=w290:u16)
                n82 = Index Array(array=w291, index=w290) -> (element=w289:T8)
                n83 = Unbundle By Name(w289) -> ("Mesh Data.Vertex Array"=w288:cluster{"X":sgl, "Y":sgl, "Z":sgl}[])
              }
            }
            n84 = Subtract(x=w280, y=w279) -> (x-y=w271:T46)
            n85 = disable-structure shown="Enabled" {
              disable-tunnel: [w306 w314] -> w272
              disable-tunnel: w271 -> [w305 w319]
              disable-tunnel: w270 -> [w304 _]
              disable-tunnel: [w302 w315] -> w269
              disable-tunnel: [_ w324] -> w268
              disable-tunnel: [_ w323] -> w267
              disable-tunnel: w266 -> [_ w322]
              disable-tunnel: w254 -> [_ w321]
              disable-tunnel: w265 -> [_ w320]
              disable-tunnel: w264 -> [_ w318]
              disable-tunnel: w263 -> [_ w317]
              disable-tunnel: w262 -> [_ w316]
              frame Disabled {
                # "Returns true if we hit the plot scene obj"
                n86 = invoke on="3D Picture Control" class="SceneGraphDisp (strict)" method="Pick Model"("Point"=w305) -> ("Pick Model"=w293:cluster{"Node Path":refnum<vi>[]}[])  [unwired: 3 in, 3 out]
                n87 = Array Size(array=w293) -> (size(s)=w294:i32)
                n88 = Unbundle By Name(w304) -> ("Fast Draw Scene Object"=w296:refnum<vi>)
                n89 = for {
                  N: w294 -> [_]
                  tunnel: w296 -> [w310]
                  tunnel: w293 -> [w308] mode=indexing
                  n90 = Unbundle(w308) -> ("Node Path"=w307:refnum<vi>[])
                  n91 = Array Size(array=w307) -> (size(s)=w309:i32)
                  n92 = for {
                    N: w309 -> [_]
                    tunnel: w307 -> [w312] mode=indexing
                    tunnel: w310 -> [w313]
                    n93 = Equal?(x=w313, y=w312) -> (x = y?=w311:bool)
                    n94 = case shown="True" w311 {
                      frame False {
                      }
                      frame True {
                      }
                    }
                  }
                }
                n95 = Index Array(array=w293, index=0) -> (element=w297:cluster{"Node Path":refnum<vi>[]})
                n96 = Unbundle(w297) -> ("Node Path"=w295:refnum<vi>[])
                n97 = Index Array(array=w295, index=1) -> (element=w300:refnum<vi>)
                n98 = Equal?(x=w296, y=w300) -> (x = y?=w299:bool)
                n99 = invoke on="3D Picture Control" class="SceneGraphDisp (strict)" method="PickPoint"("PickPoint"=w305) -> ("PickPoint"=w306:T54, "Hit"=w303:bool)  [unwired: 4 in, 3 out]
                n100 = And(x=w299, y=w303) -> (x .and. y?=w302:bool)
              }
              frame Enabled {
                n101 = call <vilib>:"pick_point.vi"("Modelview Matrix"=w322, "Projection Matrix"=w316, "Vertex Array"=w321, "Translate By"=w317, "Scale By"=w318, "Point"=w319, "ContentBounds"=w320) -> ("Hit Any Point?"=w315:bool, "Actual Ouput Coordinate"=w314:T40, "Up Vect"=w323:T40, "Forward Vect"=w324:T40)  [unwired: 1 out]
              }
            }
            n102 = case shown="True" w269 {
              tunnel: w270 -> [w329 w354]
              tunnel: [w329 w340] -> w278
              tunnel: w272 -> [_ w352]
              tunnel: w255 -> [w328 w346]
              tunnel: [w328 w346] -> w277
              tunnel: w276 -> [w327 w345]
              tunnel: w253 -> [_ w343]
              tunnel: w256 -> [w326 w341]
              tunnel: [w326 w335] -> w275
              tunnel: [w327 w342] -> w274
              tunnel: [_ TRUE] -> w273
              tunnel: w267 -> [_ w337]
              tunnel: w268 -> [_ w336]
              tunnel: w252 -> [w325 w331]
              tunnel: [w325 w330] -> w251
              frame False {
              }
              frame True {
                # "Update the cursor position and update the scene accordingly."
                n103 = Unbundle(w352) -> ("X"=w351:sgl, "Y"=w350:sgl, "Z"=w349:sgl)
                n104 = Unbundle By Name(w341) -> ("Plot/Axes/Cursor Properties.Cursor Properties Array"=w348:T29)
                n105 = Index Array(array=w348, index=w346) -> (element=w353:T53)
                n106 = Bundle By Name(cluster=w353, "Cursor Position.Position X"=w351, "Cursor Position.Position Y"=w350, "Cursor Position.Position Z"=w349) -> (w347:T53)
                n107 = Bundle By Name(cluster=w345, "Forward Vect"=w336, "Up Vect"=w337) -> (w342:T39)
                n108 = Replace Array Subset(array=w348, new element=w347, index=w346) -> (w344:T29)
                n109 = Bundle By Name(cluster=w341, "Plot/Axes/Cursor Properties.Cursor Properties Array"=w344) -> (w335:T11)
                n110 = Unbundle By Name(w335) -> ("Plot/Axes/Cursor Properties"=w334:T13, "Graph Properties"=w333:T12)
                n111 = call <vilib>:"make_scene_main.vi"("All Properties"=w334, "Scene Objects In"=w354, "Graph Properties"=w333, "Plot Processed Data"=w343, "Update?"=T43 {"Update Plot"=enum."Nothing", "Update Grid"=enum."Nothing", "Update Cursor"=enum."Update & Add", "Update Fast Draw"=enum."Nothing"}, "Track Eye"=w342) -> ("Scene Objects Out"=w340:T52)  [unwired: 9 out]
                n112 = Bundle By Name(cluster=w331, "State Changed?"=TRUE) -> (w330:T10)
              }
            }
          }
        }
      }
      event Data Change {
        # "prep VIs"
        # "Data has been changed; update everything except the cursor."
        n113 = event-data() -> ()  [unwired: 2 out]
        n114 = Unbundle By Name(w371) -> ("Plot/Axes/Cursor Properties.Plot Properties Array"=w375:T14)
        n115 = for {
          tunnel: "Data In" -> [w417] mode=indexing
          tunnel: [w416] -> w374 mode=indexing
          shift-right: [w415] -> w372
          shift-left: T6 {"Plot Rep Arrays"=[], "Graph Range Min/Max"={"X"={"Min"=0.0, "Max"=0.0}, "Y"={"Min"=0.0, "Max"=0.0}, "Z"={"Min"=0.0, "Max"=0.0}, "Amplitude"={"Min"=0.0, "Max"=0.0}}} ("Plot processed Data Out") -> [w414]
          tunnel: w375 -> [w412]
          i -> [w413]
          n116 = Array Size(array=w412) -> (size(s)=w411:i32)
          n117 = Greater Or Equal?(x=w413, y=w411) -> (x >= y?=w410:bool)
          n118 = Index Array(array=w412, index=w413) -> (element=w409:T15)
          n119 = case shown="True" w410 {
            tunnel: w409 -> [w419 _]
            tunnel: [w418 enum16{"Cartesian", "Cylindrical", "Spherical"}."Cartesian" ("Coordinate System")] -> w408
            frame False {
              n120 = Unbundle By Name(w419) -> ("Coordinate System"=w418:enum16{"Cartesian", "Cylindrical", "Spherical"})
            }
            frame True {
            }
          }
          n121 = call-dynamic "prep.vi"("Coordinate System"=w408, "Plot processed data In"=w414, "Base Datatype in"=w417) -> ("Plot processed Data Out"=w415:T6, "Base Datatype out"=w416:refnum<class "Base Datatype.lvclass">)  [unwired: 1 in, 6 out]
        }
        "Data Out" <- w374
        n122 = call <vilib>:"grow_prop_array.vi"("Display State In"=w371, "Plot processed data In"=w372) -> ("State Changed"=w369:bool, "Display State Out"=w367:T11, "Plot processed data Out"=w370:T6)  [unwired: 7 out]
        n123 = Unbundle By Name(w367) -> ("Plot/Axes/Cursor Properties"=w390:T13, "Graph Properties"=w394:T12)
        n124 = Unbundle By Name(w370) -> ("Graph Range Min/Max"=w391:T3)
        n125 = Unbundle By Name(w390) -> ("Axes Properties.from/to cluster"=w388:T3, "Axes Properties.Auto Range On"=w392:T28, "Axes Properties.Ticks Properties.Major Count"=w362:cluster{"X":i32, "Y":i32, "Z":i32}, "Format strings"=w361:T35, "Value Pair Properties"=w360:T21)
        n126 = local read "Last Axis output cluster"() -> (w359:T1)
        n127 = call <vilib>:"axes_auto_range.vi"("Acutal Range"=w391, "Auto Range On"=w392, "Set Range To"=w388) -> ("Range Min/Max"=w363:T3)  [unwired: 8 out]
        n128 = Bundle By Name(cluster=w367, "Plot/Axes/Cursor Properties.Axes Properties.from/to cluster"=w363) -> (w389:T11)
        n129 = call <vilib>:"make_value_pairs.vi"("Value Pair Properties"=w360, "Format strings"=w361, "Ticks Properties.Major Count"=w362, "Range Min/Max"=w363) -> ("Axis output cluster"=w356:T1)  [unwired: 1 in, 6 out]
        n130 = call <vilib>:"scale_names_match.vi"("Last Axis output cluster"=w359, "Axis output cluster"=w356) -> ("result"=w358:bool)  [unwired: 9 in]
        n131 = case shown="False" w358 {
          tunnel: [T43 {"Update Plot"=enum."Update & Add", "Update Grid"=enum."Update & Add", "Update Cursor"=enum."Update & Add", "Update Fast Draw"=enum."Update & Not Add"} ("Update?") T43 {"Update Plot"=enum."Update & Add", "Update Grid"=enum."Nothing", "Update Cursor"=enum."Update & Add", "Update Fast Draw"=enum."Update & Not Add"} ("Update?")] -> w357
          tunnel: w356 -> [w405 _]
          frame False {
            n132 = local write "Last Axis output cluster"(w405) -> ()
          }
          frame True {
          }
        }
        n133 = call <vilib>:"make_scene_main.vi"("All Properties"=w390, "Scene Objects In"=w355, "Graph Properties"=w394, "Plot Processed Data"=w370, "Update?"=w357, "Track Eye"=w397) -> ("Scene Objects Out"=w393:T52, "Translate By"=w402:T40, "Scale By"=w401:T40)  [unwired: 7 out]
        n134 = Equal?(x=w388, y=w363) -> (x = y?=w384:T55)
        n135 = Unbundle By Name(w384) -> ("X"=w385:cluster{"Min":bool, "Max":bool}, "Y"=w383:cluster{"Min":bool, "Max":bool}, "Z"=w382:cluster{"Min":bool, "Max":bool})
        n136 = Unbundle By Name(w385) -> ("Min"=w381:bool, "Max"=w380:bool)
        n137 = Unbundle By Name(w383) -> ("Min"=w379:bool, "Max"=w378:bool)
        n138 = Unbundle By Name(w382) -> ("Min"=w377:bool, "Max"=w376:bool)
        n139 = Compound Arithmetic op=AND(w381, w380, w379, w378, w377, w376) -> (w366:bool)
        n140 = Not(x=w366) -> (.not. x?=w365:bool)
        n141 = Or(x=w365, y=w369) -> (x .or. y?=w368:bool)
        n142 = case shown="True" w368 {
          tunnel: w387 -> [w421 w423]
          tunnel: [w421 w422] -> w386
          frame False {
          }
          frame True {
            n143 = Bundle By Name(cluster=w423, "State Changed?"=TRUE) -> (w422:T10)
          }
        }
      }
      event "3D Picture Control": Mouse Down? {
        n144 = event-data() -> ("PlatMods"=w429:T56, "Button"=w430:u16, "Coords"=w437:T46)  [unwired: 1 out]
        n145 = property on="3D Picture Control" class="SceneGraphDisp (strict)"() -> ("ContentBounds"=w446:T51, "ContentPosition"=w445:T46)  [unwired: 2 in, 2 out]
        n146 = case shown="1" w430 {
          tunnel: w429 -> [_ _ _]
          tunnel: w437 -> [w455 w474 w510]
          tunnel: [w455 w474 T46 {"Horizontal"=0, "Vertical"=0} ("Coords")] -> w441
          tunnel: w447 -> [w459 w473 _]
          tunnel: [w459 w473 w508] -> w439
          tunnel: w444 -> [_ _ w491]
          tunnel: w443 -> [_ _ w492]
          tunnel: w446 -> [_ _ w494]
          tunnel: w445 -> [_ _ w509]
          tunnel: w442 -> [_ _ w493]
          tunnel: w448 -> [w458 w472 w506]
          tunnel: [w458 w472 w501] -> w440
          tunnel: w438 -> [w456 w465 w487]
          tunnel: w436 -> [w457 w461 w498]
          tunnel: w435 -> [_ w464 w497]
          tunnel: [w457 w462 w495] -> w434
          tunnel: [_ w470 w496] -> w433
          tunnel: w432 -> [_ _ w490]
          tunnel: [_ FALSE TRUE] -> w431
          tunnel: [w456 w469 w487] -> w428
          tunnel: [_ w463 _] -> w425
          frame 0, Default {
            (unwired) T46 {"Horizontal"=0, "Vertical"=0} ("Coords")
          }
          frame 1 {
            # "We only want to use the event zoom if we are in orthographic mode.  The Perspective Zoom is already handled natively."
            # "Button 1 changes the states for fast draw"
            n147 = Unbundle By Name(w465) -> ("Graph Properties.Fast Draw"=w471:bool)
            n148 = Unbundle By Name(w465) -> ("Graph Properties.View Direction"=w466:T45)
            n149 = case shown="True" w471 {
              tunnel: w465 -> [_ w483]
              tunnel: w464 -> [_ w481]
              tunnel: [w475 w480] -> w462
              tunnel: [_ TRUE] -> w470
              tunnel: w461 -> [w475 w476]
              frame False {
              }
              frame True {
                n150 = Unbundle By Name(w483) -> ("Plot/Axes/Cursor Properties"=w482:T13, "Graph Properties"=w477:T12)
                n151 = call <vilib>:"make_scene_main.vi"("All Properties"=w482, "Scene Objects In"=w476, "Graph Properties"=w477, "Plot Processed Data"=w481, "Update?"=T43 {"Update Plot"=enum."Remove ", "Update Grid"=enum."Add", "Update Cursor"=enum."Remove ", "Update Fast Draw"=enum."Add"}) -> ("Scene Objects Out"=w480:T52)  [unwired: 1 in, 9 out]
              }
            }
            n152 = Not Equal?(x=w466, y=T45."User Define") -> (x != y?=w463:bool)
            n153 = Bundle By Name(cluster=w465, "Graph Properties.View Direction"=T45."User Define") -> (w469:T11)
          }
          frame 3 {
            # "Check if we hit a cursor when mouse button 3 is clicked.  This is done by casting a ray and testing the ray against all the cursors currently in the scene.  If the ray hits a cursor, we store the cursor's id and set \"Tracking Cursor\" to true."
            # "We only allow the cursor to move if it is visible and enabled."
            n154 = Unbundle By Name(w487) -> ("Plot/Axes/Cursor Properties.Cursor Properties Array"=w488:T29)
            n155 = disable-structure shown="Enabled" {
              disable-tunnel: w510 -> [w527 w574]
              disable-tunnel: w509 -> [w526 w575]
              disable-tunnel: [w524 w569] -> w500
              disable-tunnel: [w523 w577] -> w499
              disable-tunnel: w487 -> [w511 w564]
              disable-tunnel: w498 -> [w515 w568]
              disable-tunnel: w497 -> [w514 w566]
              disable-tunnel: [w513 w565] -> w496
              disable-tunnel: [w512 w567] -> w495
              disable-tunnel: w488 -> [_ w578]
              disable-tunnel: w494 -> [_ w576]
              disable-tunnel: w493 -> [_ w573]
              disable-tunnel: w492 -> [_ w572]
              disable-tunnel: w491 -> [_ w571]
              disable-tunnel: w490 -> [_ w570]
              frame Disabled {
                # "Button 3 is for moving cursors"
                n156 = Unbundle By Name(w515) -> ("Cursor Scene Object"=w522:refnum<vi>)
                n157 = Unbundle By Name(w511) -> ("Graph Properties.Fast Draw"=w516:bool)
                n158 = Subtract(x=w527, y=w526) -> (x-y=w525:T46)
                n159 = invoke class="SceneObject" method="Object.Object Count"(reference=w522) -> (reference out=w521:refnum<vi>, "Child Count"=w520:i32)  [unwired: 2 in, 1 out]
                n160 = invoke on="3D Picture Control" class="SceneGraphDisp (strict)" method="Pick Model"("Point"=w525) -> ("Pick Model"=w518:cluster{"Node Path":refnum<vi>[]}[])  [unwired: 3 in, 3 out]
                n161 = case shown="True" w516 {
                  tunnel: w511 -> [_ w535]
                  tunnel: w515 -> [w528 w531]
                  tunnel: [w528 w533] -> w512
                  tunnel: [_ TRUE] -> w513
                  tunnel: w514 -> [_ w529]
                  frame False {
                  }
                  frame True {
                    n162 = Unbundle By Name(w535) -> ("Plot/Axes/Cursor Properties"=w534:T13)
                    n163 = call <vilib>:"make_scene_main.vi"("All Properties"=w534, "Scene Objects In"=w531, "Plot Processed Data"=w529, "Update?"=T43 {"Update Plot"=enum."Remove ", "Update Grid"=enum."Remove ", "Update Cursor"=enum."Nothing", "Update Fast Draw"=enum."Add"}) -> ("Scene Objects Out"=w533:T52)  [unwired: 9 in, 2 out]
                  }
                }
                n164 = Array Size(array=w518) -> (size(s)=w517:i32)
                n165 = while {
                  tunnel: [w546] -> w523
                  tunnel: w521 -> [w544]
                  tunnel: w520 -> [w543]
                  tunnel: w518 -> [w542] mode=indexing
                  shift-right: [w537] -> w524
                  shift-left: FALSE -> [w541]
                  tunnel: w517 -> [w539]
                  i -> [w540]
                  stop <- w536 stop-if-true
                  n166 = Unbundle(w542) -> ("Node Path"=w545:refnum<vi>[])
                  n167 = Greater Or Equal?(x=w540, y=w539) -> (x >= y?=w538:bool)
                  n168 = Index Array(array=w545, index=2) -> (element=w548:refnum<vi>)
                  n169 = for {
                    N: w543 -> [_]
                    tunnel: w544 -> [w558]
                    tunnel: w548 -> [w557]
                    shift-right: [w555] -> w537
                    shift-left: w541 -> [w556]
                    shift-right: [w553] -> w546
                    shift-left: -1 -> [w552]
                    i -> [w554]
                    n170 = invoke class="SceneObject" method="Object.Get Object"(reference=w558, "Child Number"=w554) -> ("Get Child"=w551:refnum<vi>)  [unwired: 2 in, 3 out]
                    n171 = Equal?(x=w557, y=w551) -> (x = y?=w550:bool)
                    n172 = case shown="True" w550 {
                      tunnel: w556 -> [w560 _]
                      tunnel: [w560 TRUE] -> w555
                      tunnel: w554 -> [_ w561]
                      tunnel: [w559 w561] -> w553
                      tunnel: w552 -> [w559 _]
                      frame False {
                      }
                      frame True {
                      }
                    }
                  }
                  n173 = Or(x=w537, y=w538) -> (x .or. y?=w536:bool)
                }
              }
              frame Enabled {
                # "Button 3 is for moving cursors"
                n174 = Unbundle By Name(w564) -> ("Graph Properties.Fast Draw"=w563:bool)
                n175 = case shown="True" w563 {
                  tunnel: w564 -> [_ w591]
                  tunnel: w568 -> [w583 w587]
                  tunnel: [w583 w589] -> w567
                  tunnel: [_ TRUE] -> w565
                  tunnel: w566 -> [_ w585]
                  frame False {
                  }
                  frame True {
                    n176 = Unbundle By Name(w591) -> ("Plot/Axes/Cursor Properties"=w590:T13, "Graph Properties"=w584:T12)
                    n177 = call <vilib>:"make_scene_main.vi"("All Properties"=w590, "Scene Objects In"=w587, "Graph Properties"=w584, "Plot Processed Data"=w585, "Update?"=T43 {"Update Plot"=enum."Remove ", "Update Grid"=enum."Remove ", "Update Cursor"=enum."Nothing", "Update Fast Draw"=enum."Add"}) -> ("Scene Objects Out"=w589:T52)  [unwired: 1 in, 9 out]
                  }
                }
                n178 = for {
                  tunnel: w578 -> [w598] mode=indexing
                  shift-right: [w592] -> w579
                  shift-left: T47 [] -> [w594]
                  n179 = Unbundle By Name(w598) -> ("Cursor Position.Position X"=w597:dbl, "Cursor Position.Position Y"=w596:dbl, "Cursor Position.Position Z"=w595:dbl)
                  n180 = Bundle("Position X"=w597, "Position Y"=w596, "Position Z"=w595) -> (w593:T57)  [unwired: 1 out]
                  n181 = Build Array (concatenate)(w594, w593) -> (w592:T58)
                }
                n182 = Subtract(x=w574, y=w575) -> (x-y=w580:T46)
                n183 = call <vilib>:"pick_point.vi"("Modelview Matrix"=w571, "Projection Matrix"=w570, "Vertex Array"=w579, "Translate By"=w572, "Scale By"=w573, "Point"=w580, "ContentBounds"=w576) -> ("Hit Any Point?"=w569:bool, "Actual Ouput Coordinate"=w581:T40)  [unwired: 1 in, 2 out]
                n184 = Search 1D Array(1D array=w579, element=w581) -> (index of element=w577:i32)  [unwired: 1 out]
              }
            }
            n185 = Index Array(array=w488, index=w499) -> (element=w505:T53)
            n186 = Unbundle By Name(w505) -> ("Cursor Enable"=w504:bool, "Cursor Visible"=w502:bool, "Cursor Position.Position Snap To"=w485:enum16{"Fixed", "Nearest Plot", "Snap to Plot"})
            n187 = Not Equal?(x=w485, y=enum16{"Fixed", "Nearest Plot", "Snap to Plot"}."Fixed" ("Cursor Position.Position Snap To")) -> (x != y?=w484:bool)
            n188 = Compound Arithmetic op=AND(w500, w504, w502, w484) -> (w503:bool)
            n189 = case shown="True" w503 {
              selector: w503 -> [w599 w602]
              tunnel: w506 -> [w600 _]
              tunnel: [w600 w601] -> w501
              tunnel: [w599 w602] -> w508
              tunnel: w499 -> [_ w601]
              frame False {
              }
              frame True {
              }
            }
          }
        }
        n190 = case shown="True" w425 {
          tunnel: w427 -> [w451 w453]
          tunnel: [w451 w452] -> w426
          frame False {
          }
          frame True {
            n191 = Bundle By Name(cluster=w453, "State Changed?"=TRUE) -> (w452:T10)
          }
        }
        n192 = event-data("Button"=w430, "PlatMods"=w429, "Discard?"=w431) -> ()  [unwired: 1 in, 1 out]
      }
      event Panel Resize {
        n193 = event-data() -> ()  [unwired: 2 out]
      }
      event "3D Picture Control": Mouse Up {
        # "Here, we check if we are doing fast draw or not.  If we are, then update all of the scene."
        # "When the Mouse is up, there is a good chance that the position of the eye has changed.  We want to change the state accordingly.  \"Pick Point\" not only picks out points but also output the forward&up vectors in world coordinates.  We use those two vectors to update any view-independent things in our scene.  Currently, the only view-independent component is the cursor text."
        n194 = event-data() -> ("Button"=w617:u16)  [unwired: 8 out]
        n195 = Unbundle By Name(w635) -> ("Plot/Axes/Cursor Properties"=w634:T13, "Graph Properties.Fast Draw"=w628:bool, "Graph Properties"=w620:T12)
        n196 = Equal?(x=w617, y=u16 1 ("x")) -> (x = y?=w622:bool)
        n197 = Equal?(x=w617, y=u16 3 ("x")) -> (x = y?=w623:bool)
        n198 = property on="3D Picture Control" class="SceneGraphDisp (strict)"() -> ("ModelView Matrix"=w619:sgl[][], "Projection Matrix"=w618:sgl[][])  [unwired: 2 in, 2 out]
        n199 = Or(x=w622, y=w623) -> (x .or. y?=w621:bool)
        n200 = And(x=w628, y=w621) -> (x .and. y?=w627:bool)
        n201 = case shown="False" w627 {
          tunnel: [T43 {"Update Plot"=enum."Nothing", "Update Grid"=enum."Update & Add", "Update Cursor"=enum."Update & Add", "Update Fast Draw"=enum."Nothing"} ("Update?") T43 {"Update Plot"=enum."Add", "Update Grid"=enum."Update & Add", "Update Cursor"=enum."Update & Add", "Update Fast Draw"=enum."Remove "} ("Update?")] -> w629
          frame False {
          }
          frame True {
          }
        }
        n202 = call <vilib>:"pick_point.vi"("Modelview Matrix"=w619, "Projection Matrix"=w618) -> ("Up Vect"=w636:T40, "Forward Vect"=w637:T40)  [unwired: 5 in, 3 out]
        n203 = Bundle By Name(cluster=T39 {"Forward Vect"={"X"=0.0, "Y"=0.0, "Z"=0.0}, "Up Vect"={"X"=0.0, "Y"=0.0, "Z"=0.0}} ("Track Eye"), "Forward Vect"=w637, "Up Vect"=w636) -> (w631:T39)
        n204 = call <vilib>:"make_scene_main.vi"("All Properties"=w634, "Scene Objects In"=w640, "Graph Properties"=w620, "Plot Processed Data"=w639, "Update?"=w629, "Track Eye"=w631) -> ("Scene Objects Out"=w630:T52)  [unwired: 9 out]
      }
      event Display State Change {
        n205 = event-data() -> ()  [unwired: 5 out]
        n206 = Unbundle By Name(w659) -> ("Disable Updates"=w658:bool)
        n207 = case shown="False" w658 {
          tunnel: w659 -> [w673 _]
          tunnel: w657 -> [w680 w732]
          tunnel: [w679 w732] -> w656
          tunnel: w649 -> [w669 w729]
          tunnel: w655 -> [w678 _]
          tunnel: w654 -> [_ w731]
          tunnel: [w677 w731] -> w653
          tunnel: [w676 w730] -> w651
          tunnel: w652 -> [_ w730]
          tunnel: w650 -> [w668 _]
          tunnel: [w667 w729] -> w648
          frame False {
            n208 = local read "Coord Systems"() -> (w674:T5)
            n209 = Unbundle By Name(w673) -> ("Plot/Axes/Cursor Properties.Plot Properties Array"=w672:T14)
            n210 = flat-sequence {
              tunnel: w680 -> [w717]
              tunnel: [w716] -> w679
              tunnel: w667 -> [w711]
              tunnel: w678 -> [w715]
              tunnel: [w714] -> w677
              tunnel: [w713] -> w676
              tunnel: w673 -> [w712]
              tunnel: w668 -> [w710]
              frame #0 {
                n211 = Unbundle By Name(w712) -> ("Plot/Axes/Cursor Properties"=w720:T13, "Graph Properties"=w719:T12)
                n212 = control-ref of="3D Picture Control"() -> (w724:refnum<vi>)
                n213 = disable-structure shown="Enabled" {
                  disable-tunnel: w719 -> [w725 _]
                  frame Enabled {
                    n214 = local read "Hardware Window Refnum"() -> (w726:refnum<vi>)
                    n215 = call <vilib>:"set_up_graph_hardware_window_properties.vi"("Graph Properties"=w725, "Hardware Window Refnum"=w726) -> ()  [unwired: 10 out]
                  }
                  frame Disabled {
                  }
                }
                n216 = call <vilib>:"set_up_graph_control_properties.vi"("Graph Properties"=w719, "viewing volume"=w710, "3D Picture Control Reference"=w724) -> ()  [unwired: 1 in, 8 out]
                n217 = call <vilib>:"make_scene_main.vi"("All Properties"=w720, "Scene Objects In"=w717, "Graph Properties"=w719, "Plot Processed Data"=w711, "Update?"=T43 {"Update Plot"=enum."Update & Add", "Update Grid"=enum."Update & Add", "Update Cursor"=enum."Update & Add", "Update Fast Draw"=enum."Update & Not Add"}, "Track Eye"=w715) -> ("Scene Objects Out"=w716:T52, "Translate By"=w713:T40, "Scale By"=w714:T40)  [unwired: 7 out]
                n218 = Unbundle By Name(w712) -> ("Graph Properties.Lighting"=w718:bool)
                n219 = case shown="False" w718 {
                  tunnel: [enum16{"Inherit Value", "Off", "On"}."Off" ("Specials:Lighting") enum16{"Inherit Value", "Off", "On"}."On" ("Specials:Lighting")] -> w722
                  frame False {
                  }
                  frame True {
                  }
                }
                n220 = Unbundle By Name(w716) -> ("Root"=w721:refnum<vi>)
                n221 = property class="SceneObject"(reference=w721, "Specials.Lighting"=w722) -> ()  [unwired: 1 in, 2 out]
              }
            }
            n222 = for {
              tunnel: w674 -> [w704]
              shift-right: [w705] -> w670
              shift-left: FALSE -> [w706]
              tunnel: [w700] -> w671 mode=indexing
              tunnel: w672 -> [w701] mode=indexing
              i -> [w703]
              n223 = Unbundle By Name(w701) -> ("Coordinate System"=w700:enum16{"Cartesian", "Cylindrical", "Spherical"})
              n224 = Index Array(array=w704, index=w703) -> (element=w702:enum16{"Cartesian", "Cylindrical", "Spherical"})
              n225 = Not Equal?(x=w702, y=w700) -> (x != y?=w707:bool)
              n226 = case shown="False" w707 {
                selector: w707 -> [_ w709]
                tunnel: w706 -> [w708 _]
                tunnel: [w708 w709] -> w705
                frame False {
                }
                frame True {
                }
              }
            }
            n227 = local write "Coord Systems"(w671) -> ()
            n228 = case shown="True" w670 {
              tunnel: [w681 w686] -> w667
              tunnel: w672 -> [_ w682]
              tunnel: w669 -> [w681 _]
              frame False {
              }
              frame True {
                n229 = local read "Data In"() -> (w684:T38)
                n230 = for {
                  tunnel: [w696] -> w683 mode=indexing
                  shift-right: [w695] -> w686
                  shift-left: T6 {"Plot Rep Arrays"=[], "Graph Range Min/Max"={"X"={"Min"=0.0, "Max"=0.0}, "Y"={"Min"=0.0, "Max"=0.0}, "Z"={"Min"=0.0, "Max"=0.0}, "Amplitude"={"Min"=0.0, "Max"=0.0}}} ("Plot processed Data Out") -> [w694]
                  tunnel: w682 -> [w687]
                  tunnel: w684 -> [w688] mode=indexing
                  i -> [w693]
                  n231 = Array Size(array=w687) -> (size(s)=w692:i32)
                  n232 = Index Array(array=w687, index=w693) -> (element=w690:T15)
                  n233 = Greater Or Equal?(x=w693, y=w692) -> (x >= y?=w691:bool)
                  n234 = case shown="True" w691 {
                    tunnel: w690 -> [w698 _]
                    tunnel: [w697 enum16{"Cartesian", "Cylindrical", "Spherical"}."Cartesian" ("Coordinate System")] -> w689
                    frame False {
                      n235 = Unbundle By Name(w698) -> ("Coordinate System"=w697:enum16{"Cartesian", "Cylindrical", "Spherical"})
                    }
                    frame True {
                    }
                  }
                  n236 = call-dynamic "prep.vi"("Coordinate System"=w689, "Plot processed data In"=w694, "Base Datatype in"=w688) -> ("Plot processed Data Out"=w695:T6, "Base Datatype out"=w696:refnum<class "Base Datatype.lvclass">)  [unwired: 1 in, 6 out]
                }
                n237 = local write "Data Out"(w683) -> ()
              }
            }
          }
          frame True {
          }
        }
      }
      event Direction Change {
        n238 = event-data() -> ()  [unwired: 2 out]
        n239 = Unbundle By Name(w746) -> ()  [unwired: 1 out]
      }
      event Exec State Change {
        n240 = event-data() -> ()  [unwired: 2 out]
        n241 = Unbundle By Name(w760) -> ()  [unwired: 1 out]
      }
    }
    n242 = case shown="True" w22 {
      frame False {
      }
      frame True {
        n243 = local read "Hardware Window Refnum"() -> (w47:refnum<vi>)
        n244 = property class="SceneWindow"(reference=w47) -> ("State"=w48:T42)  [unwired: 1 in, 2 out]
        n245 = case shown="\"Open\", Default" w48 {
          tunnel: w47 -> [w49 _]
          frame "Open", Default {
            n246 = invoke class="SceneWindow" method="Redraw"(reference=w49) -> ()  [unwired: 2 in, 3 out]
          }
          frame "Minimized" {
          }
        }
        n247 = invoke on="3D Picture Control" class="SceneGraphDisp (strict)" method="Redraw"() -> ()  [unwired: 3 in, 3 out]
      }
    }
  }
  "Display State Out" <- w3
  "Action" <- w4
  "Plot processed data out" <- w6
